vi "TSM Initialise Global (Process Setup).vi"(0 "TSM context":T2, 5 "TestFlowID":string, 9 "configuration file path":string) -> (4 "Initial Configurations":T1, 15 "error out":errorcluster)   [LabVIEW 2019]
uses:
  <vilib>/NI_TestStand_SemiconductorModule/NI_TestStand_Semiconductor_Module.lvlibp/PinMap/General/SemiconductorModuleContext.ctl
  Common/Utility/typedefs/Initial Configurations.ctl
  Common/Instrument Control/DCPower/TSM/TSM SSC DCPower.ctl
  <vilib>/NI_TestStand_SemiconductorModule/NI_TestStand_Semiconductor_Module.lvlibp/PinMap/PinQueryContext/MultiplePinMultipleSessionQueryContext/MultiplePinMultipleSessionQueryContext.lvclass
  Common/Instrument Control/DCPower/SSC DCPower/SSC DCPower.ctl
  Common/Instrument Control/Shared SubVIs/TSM Pin Abstraction/TSM Pin Information.ctl
  Common/Instrument Control/Shared SubVIs/TSM Pin Abstraction/TSM Pin Type Identifier.ctl
  Common/Instrument Control/Shared SubVIs/TSM Pin Abstraction/TSM Expanded Pin Information.ctl
  Common/Instrument Control/Relay/Pin Map/TSM Relay.ctl
  Common/Instrument Control/DAQmx/Pin Map/TSM DAQmx Multi-Task.ctl
  Common/Instrument Control/DAQmx/Pin Map/SSC DAQmx.ctl
  TSM Context Data Access/TSM Context Data Access.lvclass/TSM Context Data Access.ctl
  TSM Context Data Access/Public/Properties/K1 - Write.vi
  TSM Context Data Access/Public/Properties/MODE3 - Write.vi
  TSM Context Data Access/Public/Properties/Z - Write.vi
  TSM Context Data Access/Public/Properties/Y - Write.vi
  TSM Context Data Access/Public/Properties/MODE2 - Write.vi
  TSM Context Data Access/Public/Properties/K1 - Read.vi
  TSM Context Data Access/Public/Properties/MODE3 - Read.vi
  TSM Context Data Access/Public/Properties/MODE2 - Read.vi
  TSM Context Data Access/Public/Properties/Z - Read.vi
  TSM Context Data Access/Public/Properties/Y - Read.vi
  TSM Context Data Access/Public/Properties/S1 - Write .vi
  TSM Context Data Access/Public/Properties/S1 - Read.vi
  TSM Context Data Access/Public/Properties/DNUM - Write.vi
  TSM Context Data Access/Public/Properties/U0 - Write.vi
  TSM Context Data Access/Public/Properties/U1 - Write.vi
  TSM Context Data Access/Public/Properties/U2- Write.vi
  TSM Context Data Access/Public/Properties/U3 - Write.vi
  TSM Context Data Access/Public/Properties/U4 - Write.vi
  TSM Context Data Access/Public/Properties/U5 - Write.vi
  TSM Context Data Access/Public/Properties/U7 - Write.vi
  TSM Context Data Access/Public/Properties/U8 - Write.vi
  TSM Context Data Access/Public/Properties/U9 - Write.vi
  TSM Context Data Access/Public/Properties/Z1 - Write.vi
  TSM Context Data Access/Public/Properties/Z2- Write.vi
  TSM Context Data Access/Public/Properties/Z3 - Write.vi
  TSM Context Data Access/Public/Properties/Z4 - Write.vi
  TSM Context Data Access/Public/Properties/Z5 - Write.vi
  TSM Context Data Access/Public/Properties/Z6 - Write.vi
  TSM Context Data Access/Public/Properties/Z7 - Write.vi
  TSM Context Data Access/Public/Properties/Z8 - Write.vi
  TSM Context Data Access/Public/Properties/Z9 - Write.vi
  TSM Context Data Access/Public/Properties/New_Global/ReferenceData - Write.vi
  TSM Context Data Access/Public/Properties/C1 - Write.vi
  TSM Context Data Access/Public/Properties/C2 - Write.vi
  TSM Context Data Access/Public/Properties/C3 - Write.vi
  TSM Context Data Access/Public/Properties/C4 - Write.vi
  TSM Context Data Access/Public/Properties/C5 - Write.vi
  TSM Context Data Access/Public/Properties/C6 - Write.vi
  TSM Context Data Access/Public/Properties/C7 - Write.vi
  TSM Context Data Access/Public/Properties/C9 - Write.vi
  <vilib>/NI_TestStand_SemiconductorModule/NI_TestStand_Semiconductor_Module.lvlibp/PinMap/Site and Global Data/SetGlobalData.vi
  TSM Context Data Access/Public/Properties/TestFlowID - Write.vi
  <vilib>/NI_TestStand_SemiconductorModule/NI_TestStand_Semiconductor_Module.lvlibp/PinMap/Site and Global Data/GetGlobalData.vi
  <vilib>/NI_TestStand_SemiconductorModule/NI_TestStand_Semiconductor_Module.lvlibp/PinMap/Site and Global Data/SetSiteData.vi
  <vilib>/NI_TestStand_SemiconductorModule/NI_TestStand_Semiconductor_Module.lvlibp
  TSM Context Data Access/TSM Context Data Access.lvclass
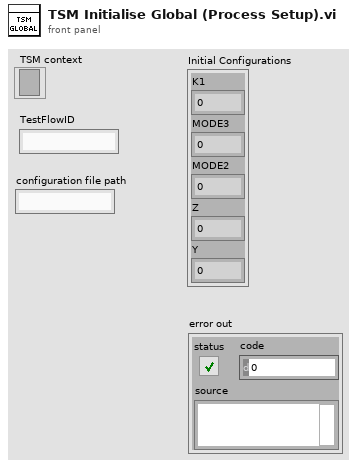
[diagram p1: front panel]
types:
  T1 = typedef "Initial Configurations.ctl" = cluster{"K1":i8, "MODE3":i8, "MODE2":i8, "Z":i8, "Y":i8}
  T2 = typedef "NI_TestStand_Semiconductor_Module.lvlibp/SemiconductorModuleContext.ctl" = refnum<k7>
  T3 = cluster{"unloaded12VRLY":dbl[], "vdiode":dbl[], "RelayDrop":dbl[][], "Initial Configurations":T1}
  T4 = typedef "TSM SSC DCPower.ctl" = cluster{"Pin Query Context":refnum<class "MultiplePinMultipleSessionQueryContext.lvclass">, "SSC":T5[], "Site Numbers":i32[], "Pins":T6[], "Pins Expanded":T8[]}
  T5 = typedef "SSC DCPower.ctl" = cluster{"Session":refnum<k15>, "Chan":string, "Channel List":string}
  T6 = typedef "TSM Pin Information.ctl" = cluster{"Pin":tag, "Type":T7, "Count":i32}
  T7 = typedef "TSM Pin Type Identifier.ctl" = enum8{"DUT Pin", "System Pin", "Pin Group", "Not Determined"}
  T8 = typedef "TSM Expanded Pin Information.ctl" = cluster{"Pin":tag, "Type":T7, "Index":i32}
  T9 = typedef "TSM Relay.ctl" = cluster{"TSM Context":T2, "Relays":tag[]}
  T10 = typedef "TSM DAQmx Multi-Task.ctl" = cluster{"Pin Query Context":refnum<class "MultiplePinMultipleSessionQueryContext.lvclass">, "SSC":T11[], "Site Numbers":i32[]}
  T11 = typedef "SSC DAQmx.ctl" = cluster{"DAQmx Task ":refnum<k21>, "Channels":string, "Channel Lists":string}
  T12 = cluster{"Number Of Sites":i32, "Site Numbers":i32[], "RLY12V_MEAS":T4, "Relays Filtered Pins":string[], "Relay Pin Sessions":T9[], "UDB_EN":T10}
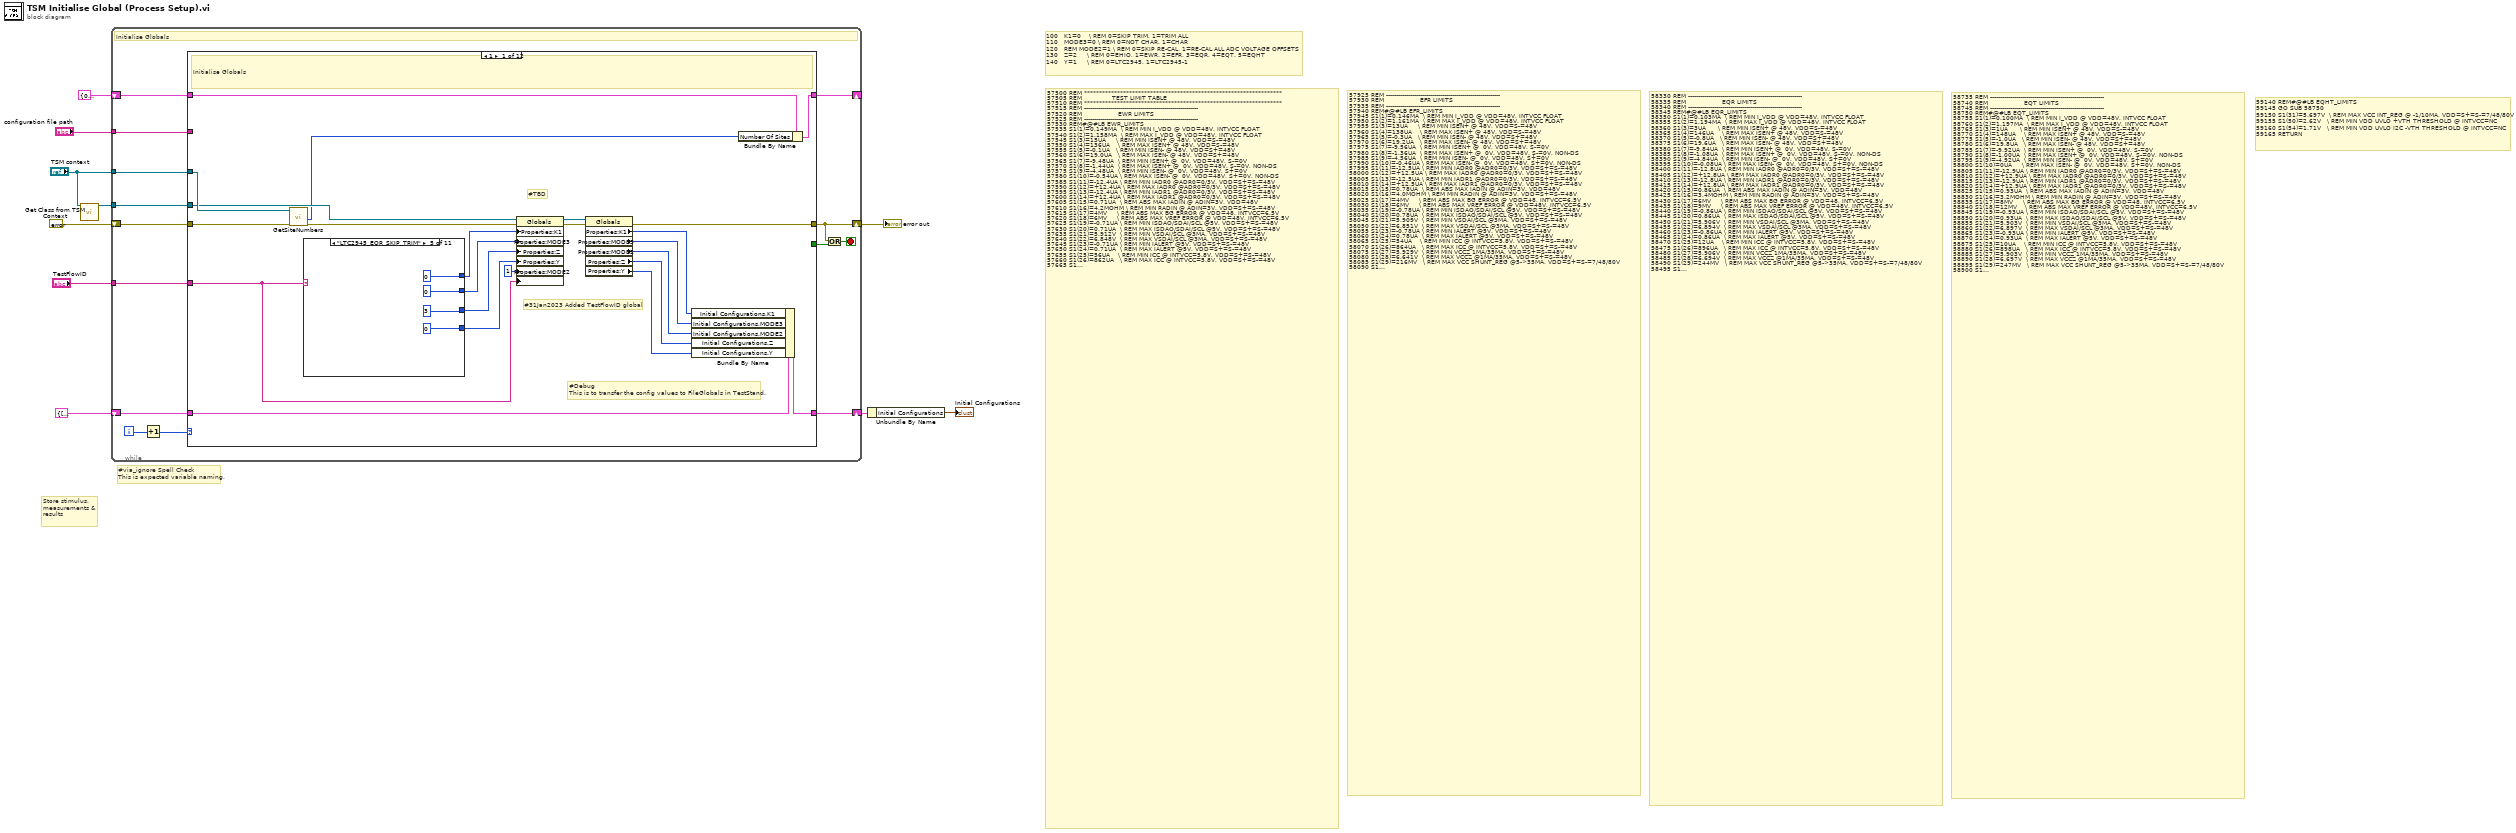
[diagram p0: block diagram]
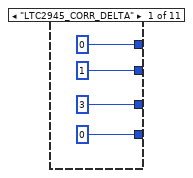
[diagram p2: hidden frame]
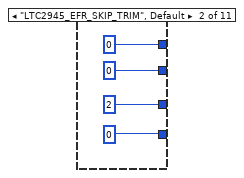
[diagram p3: hidden frame]
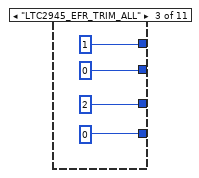
[diagram p4: hidden frame]
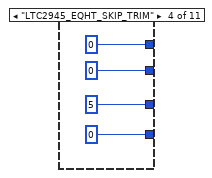
[diagram p5: hidden frame]
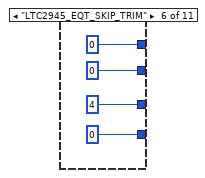
[diagram p6: hidden frame]
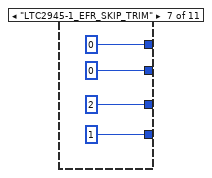
[diagram p7: hidden frame]
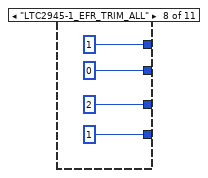
[diagram p8: hidden frame]
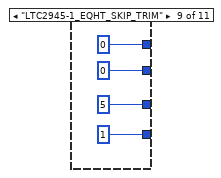
[diagram p9: hidden frame]
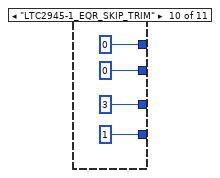
[diagram p10: hidden frame]
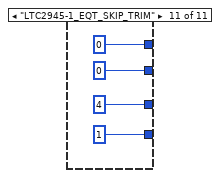
[diagram p11: hidden frame]
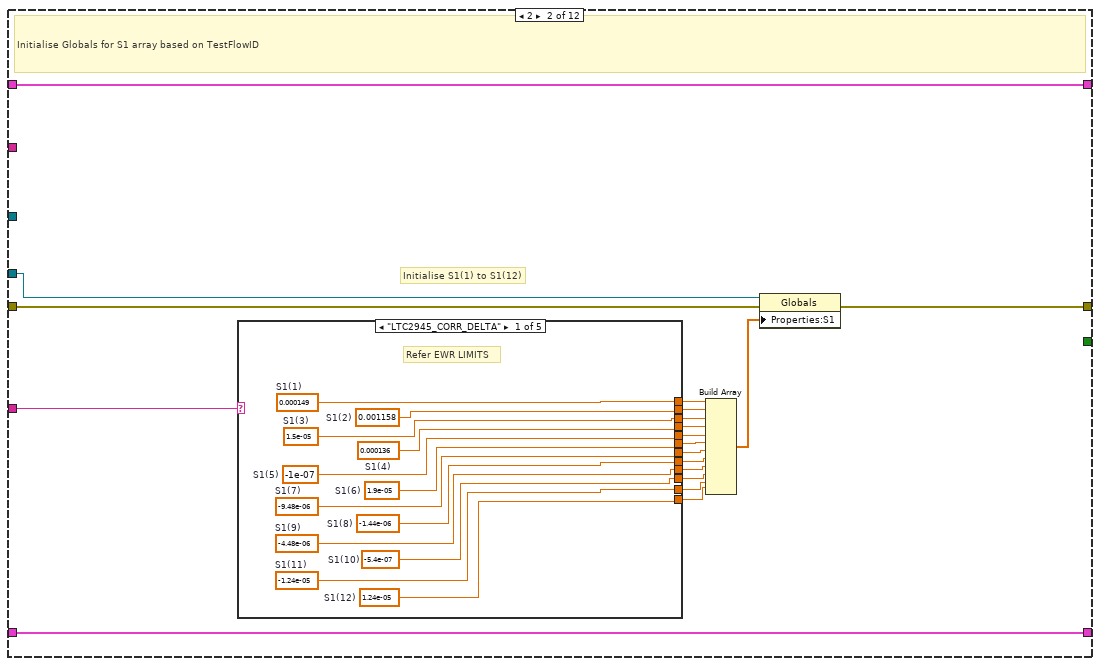
[diagram p12: hidden frame]
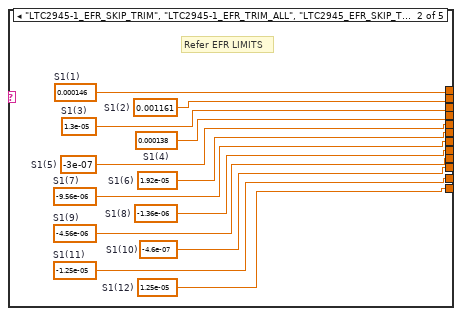
[diagram p13: hidden frame]
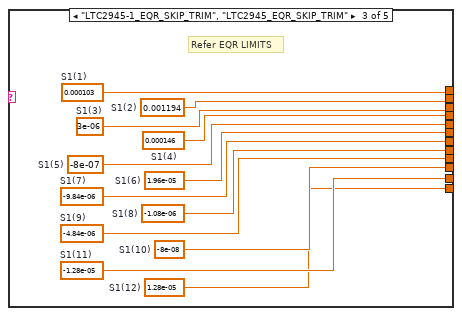
[diagram p14: hidden frame]
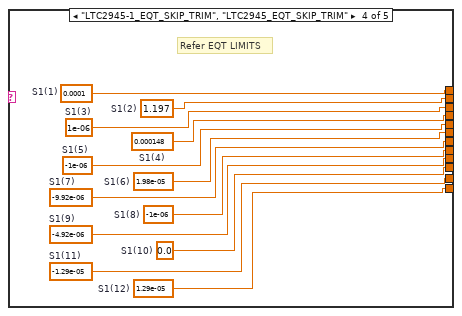
[diagram p15: hidden frame]
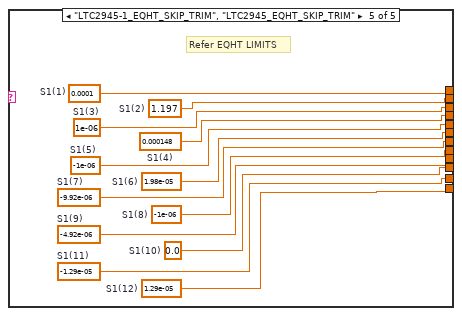
[diagram p16: hidden frame]
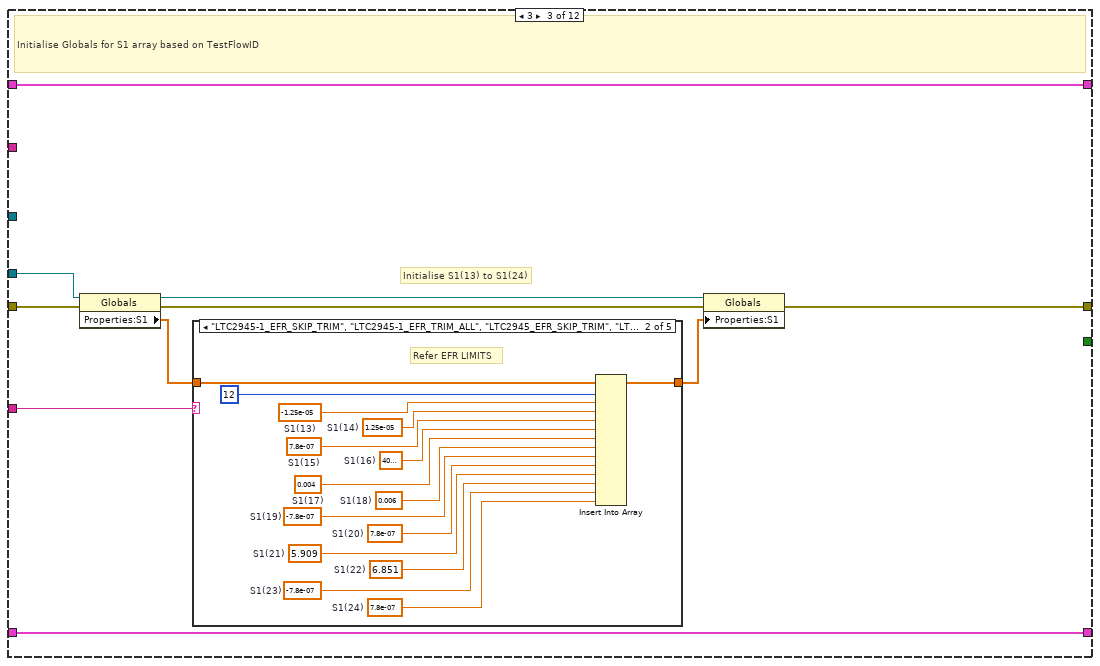
[diagram p17: hidden frame]
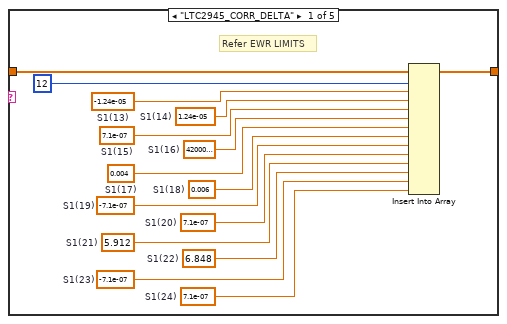
[diagram p18: hidden frame]
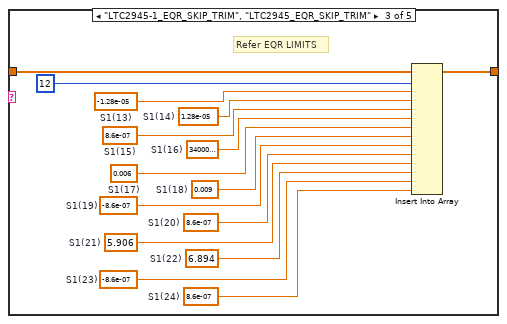
[diagram p19: hidden frame]
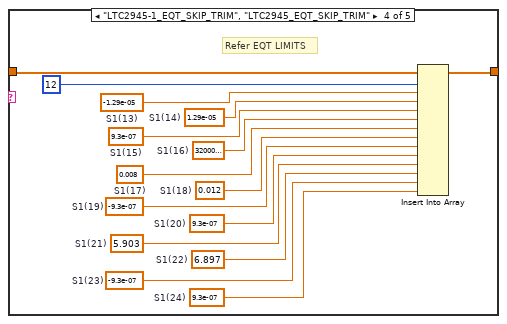
[diagram p20: hidden frame]
diagram:
  # "59140 REM#@#LB EQHT_LIMITS\n59145 GO SUB 58750\n59150 S1(31)=5.697V  \\ REM MAX VCC INT_REG @ -1/10MA, VDD=S+=S-=7/48/80V\n59155 S1(50)=2.62V   \\ REM MIN VDD UVLO +VTH THRESHOLD @ INTVCC=NC\n59160 S1(54)=1.71V   \\ REM MIN VDD UVLO I2C -VTH THRESHOLD @ INTVCC=NC\n59165 RETURN"
  # "58735 REM ---------------------------------------------------------\n58740 REM                  EQT LIMITS\n58745 REM ---------------------------------------------------------\n58750 REM#@#LB EQT_LIMITS\n58755 S1(1)=0.100MA  \\ REM MIN I_VDD @ VDD=48V, INTVCC FLOAT\n58760 S1(2)=1.197MA  \\ REM MAX I_VDD @ VDD=48V, INTVCC FLOAT\n58765 S1(3)=1UA      \\ REM MIN ISEN+ @ 48V, VDD=S-=48V\n58770 S1(4)=148UA    \\ REM MAX ISEN+ @ 48V, VDD=S-=48V\n58775 S1(5)=-1.0UA   \\ REM MIN ISEN- @ 48V, VDD=S+=48V\n58780 S1(6)=19.8UA   \\ REM MAX ISEN- @ 48V, VDD=S+=48V\n58785 S1(7)=-9.92UA  \\ REM MIN ISEN+ @  0V, VDD=48V, S-=0V\n58790 S1(8)=-1.00UA  \\ REM MAX ISEN+ @  0V, VDD=48V, S-=0V, NON-DS\n58795 S1(9)=-4.92UA  \\ REM MIN ISEN- @  0V, VDD=48V, S+=0V\n58800 S1(10)=0UA     \\ REM MAX ISEN- @  0V, VDD=48V, S+=0V, NON-DS\n58805 S1(11)=-12.9UA \\ REM MIN IADR0 @ADR0=0/3V, VDD=S+=S-=48V\n58810 S1(12)=+12.9UA \\ REM MAX IADR0 @ADR0=0/3V, VDD=S+=S-=48V\n58815 S1(13)=-12.9UA \\ REM MIN IADR1 @ADR0=0/3V, VDD=S+=S-=48V\n58820 S1(14)=+12.9UA \\ REM MAX IADR1 @ADR0=0/3V, VDD=S+=S-=48V\n58825 S1(15)=0.93UA  \\ REM ABS MAX IADIN @ ADIN=3V, VDD=48V\n58830 S1(16)=3.2MOHM \\ REM MIN RADIN @ ADIN=3V, VDD=S+=S-=48V\n58835 S1(17)=8MV     \\ REM ABS MAX BG ERROR @ VDD=48, INTVCC=6.5V\n58840 S1(18)=12MV    \\ REM ABS MAX VREF ERROR @ VDD=48V, INTVCC=6.5V\n58845 S1(19)=-0.93UA \\ REM MIN ISDAO/SDAI/SCL @5V, VDD=S+=S-=48V\n58850 S1(20)=0.93UA  \\ REM MAX ISDAO/SDAI/SCL @5V, VDD=S+=S-=48V\n58855 S1(21)=5.903V  \\ REM MIN VSDAI/SCL @3MA, VDD=S+=S-=48V\n58860 S1(22)=6.897V  \\ REM MAX VSDAI/SCL @3MA, VDD=S+=S-=48V\n58865 S1(23)=-0.93UA \\ REM MIN IALERT @5V, VDD=S+=S-=48V\n58870 S1(24)=0.93UA  \\ REM MAX IALERT @5V, VDD=S+=S-=48V\n58875 S1(25)=10UA    \\ REM MIN ICC @ INTVCC=5.8V, VDD=S+=S-=48V\n58880 S1(26)=898UA   \\ REM MAX ICC @ INTVCC=5.8V, VDD=S+=S-=48V\n58885 S1(27)=5.903V  \\ REM MIN VCCZ 1MA/35MA, VDD=S+=S-=48V\n58890 S1(28)=6.697V  \\ REM MAX VCCZ @1MA/35MA, VDD=S+=S-=48V\n58895 S1(29)=247MV   \\ REM MAX VCC SHUNT_REG @5->35MA, VDD=S+=S-=7/48/80V\n58900 S1(30)=4.503V  \\ REM MIN VCC INT_REG @ -1/10MA, VDD=S+=S-=7/48/80V\n58905 S1(31)=5.497V  \\ REM MAX VCC INT_REG @ -1/10MA, VDD=S+=S-=7/48/80V\n58910 S1(32)=198MV   \\ REM MAX VCC LOAD REG @1->10MA, VDD=S+=S-=7/48/80V\n58915 S1(33)=1.92UA  \\ REM MAX ISEN+ SHDN @ 0/48V, VDD=S-=48V\n58920 S1(34)=0.92UA  \\ REM MAX ISEN- SHDN @ 0/48V, VDD=48V, S-=0V\n58925 S1(35)=79UA    \\ REM MAX ICC_SD @ INTVCC=5V, VDD=S+=S-=48V\n58930 S1(36)=69UA    \\ REM MAX IDD_SD @ INTVCC=NC, S+=S-=48V\n58935 S1(37)=0.73%   \\ REM ABS MAX ADC DELTA VSENSE T.U.E, VDD=4/48/80V\n58940 S1(38)=0.73%   \\ REM ABS MAX ADC ADIN T.U.E, VDD=4/48/80V, S+=48V\n58945 S1(39)=0.73%   \\ REM ABS MAX ADC VIN (VDD&S+) T.U.E, S+=48V\n58950 S1(40)=1.92V   \\ REM MIN ADR0/AD1 VIH @ VDD=48V\n58955 S1(41)=2.68V   \\ REM MAX ADR0/AD1 VIH @ VDD=48V\n58960 S1(42)=0.32V   \\ REM MIN ADR0/AD1 VIL @ VDD=48V\n58965 S1(43)=0.88V   \\ REM MAX ADR0/AD1 VIL @ VDD=48V\n58970 S1(44)=10MV    \\ REM MIN SDAO/ALERT VOL @8MA, VDD=48V\n58975 S1(45)=398MV   \\ REM MAX SDAO/ALERT VOL @8MA, VDD=48V\n58980 S1(46)=1.52V   \\ REM MIN SDAI/SCL VTH @ VDD=48V\n58985 S1(47)=2.18V   \\ REM MAX SDAI/SCL VTH @ VDD=48V\n58990 S1(48)=2.31V   \\ REM MIN VCC UVLO +VTH THRESHOLD @ VDD=INTVCC\n58995 S1(49)=2.68V   \\ REM MAX VCC UVLO +VTH THRESHOLD @ VDD=INTVCC\n59000 S1(50)=2.92V   \\ REM MIN VDD UVLO +VTH THRESHOLD @ INTVCC=NC\n59005 S1(51)=3.48V   \\ REM MAX VDD UVLO +VTH THRESHOLD @ INTVCC=NC\n59010 S1(52)=1.51V   \\ REM MIN VCC UVLO I2C -VTH THRESHOLD @ VDD=INTVCC\n59015 S1(53)=2.60V   \\ REM MAX VCC UVLO I2C +VTH THRESHOLD @ VDD=INTVCC (NON-DS)\n59020 S1(54)=2.01V   \\ REM MIN VDD UVLO I2C -VTH THRESHOLD @ INTVCC=NC\n59025 S1(55)=3.20V   \\ REM MAX VDD UVLO I2C +VTH THRESHOLD @ INTVCC=NC, (NON-DS)\n59030 S1(59)=25MS    \\ REM STUCK BUS MIN TIMING\n59035 S1(60)=50MS    \\ REM STUCK BUS MAX TIMING\n59040 S1(61)=0.20MA  \\ REM MIN ABSMAX I_VDD @ VDD=90/100V\n59045 S1(62)=2.00MA  \\ REM MAX ABSMAX I_VDD @ VDD=90/100V\n59050 S1(63)=1UA     \\ REM MIN ABSMAX ISEN+ @ VSEN+=100V\n59055 S1(64)=200UA   \\ REM MAX ABSMAX ISEN+ @ VSEN+=100V\n59060 S1(65)=-0.2UA  \\ REM MIN ABSMAX ISEN- @ VSEN-=100V\n59065 S1(66)=40UA    \\ REM MAX ABSMAX ISEN- @ VSEN-=100V\n59070 S1(67)=2.99LSB \\ REM ABS MAX ADC DELTA VSENSE INL ERROR, VDD=2.7V\n59075 S1(68)=1.99LSB \\ REM ABS MAX ADC ADIN INL ERROR, VDD=4/48/80V, S+=48V\n59080 S1(69)=1.99LSB \\ REM ABS MAX ADC VIN (VDD&S+) INL ERROR, S+=48V\n59085 S1(70)=3.09LSB \\ REM ABS MAX ADC DELTA VSENSE VOS, VDD=2.7V\n59090 S1(71)=1.09LSB \\ REM ABS MAX ADC ADIN VOS, VDD=2.7V\n59095 S1(72)=1.49LSB \\ REM ABS MAX ADC VIN (VDD&S+) VOS, S+=48V\n59100 S1(73)=30.01MS \\ REM MIN VIN/ADIN CONVERSION TIME @ VDD=S+=S-=48V\n59105 S1(74)=35.99MS \\ REM MAX VIN/ADIN CONVERSION TIME @ VDD=S+=S-=48V\n59110 S1(75)=60.02MS \\ REM MIN DVSENSE CONVERSION TIME @ VDD=S+=S-=48V\n59115 S1(76)=71.98MS \\ REM MAX DVSENSE CONVERSION TIME @ VDD=S+=S-=48V\n59120 S1(77)=6.01HZ  \\ REM MIN CONVERSION RATE @ VDD=S+=S-=48V\n59125 S1(78)=8.99HZ  \\ REM MAX CONVERSION RATE @ VDD=S+=S-=48V\n59130 Z0=1\n59135 RETURN"
  # "58330 REM ---------------------------------------------------------\n58335 REM                  EQR LIMITS\n58340 REM ---------------------------------------------------------\n58345 REM#@#LB EQR_LIMITS\n58350 S1(1)=0.103MA  \\ REM MIN I_VDD @ VDD=48V, INTVCC FLOAT\n58355 S1(2)=1.194MA  \\ REM MAX I_VDD @ VDD=48V, INTVCC FLOAT\n58360 S1(3)=3UA      \\ REM MIN ISEN+ @ 48V, VDD=S-=48V\n58365 S1(4)=146UA    \\ REM MAX ISEN+ @ 48V, VDD=S-=48V\n58370 S1(5)=-0.8UA   \\ REM MIN ISEN- @ 48V, VDD=S+=48V\n58375 S1(6)=19.6UA   \\ REM MAX ISEN- @ 48V, VDD=S+=48V\n58380 S1(7)=-9.84UA  \\ REM MIN ISEN+ @  0V, VDD=48V, S-=0V\n58385 S1(8)=-1.08UA  \\ REM MAX ISEN+ @  0V, VDD=48V, S-=0V, NON-DS\n58390 S1(9)=-4.84UA  \\ REM MIN ISEN- @  0V, VDD=48V, S+=0V\n58395 S1(10)=-0.08UA \\ REM MAX ISEN- @  0V, VDD=48V, S+=0V, NON-DS\n58400 S1(11)=-12.8UA \\ REM MIN IADR0 @ADR0=0/3V, VDD=S+=S-=48V\n58405 S1(12)=+12.8UA \\ REM MAX IADR0 @ADR0=0/3V, VDD=S+=S-=48V\n58410 S1(13)=-12.8UA \\ REM MIN IADR1 @ADR0=0/3V, VDD=S+=S-=48V\n58415 S1(14)=+12.8UA \\ REM MAX IADR1 @ADR0=0/3V, VDD=S+=S-=48V\n58420 S1(15)=0.86UA  \\ REM ABS MAX IADIN @ ADIN=3V, VDD=48V\n58425 S1(16)=3.4MOHM \\ REM MIN RADIN @ ADIN=3V, VDD=S+=S-=48V\n58430 S1(17)=6MV     \\ REM ABS MAX BG ERROR @ VDD=48, INTVCC=6.5V\n58435 S1(18)=9MV     \\ REM ABS MAX VREF ERROR @ VDD=48V, INTVCC=6.5V\n58440 S1(19)=-0.86UA \\ REM MIN ISDAO/SDAI/SCL @5V, VDD=S+=S-=48V\n58445 S1(20)=0.86UA  \\ REM MAX ISDAO/SDAI/SCL @5V, VDD=S+=S-=48V\n58450 S1(21)=5.906V  \\ REM MIN VSDAI/SCL @3MA, VDD=S+=S-=48V\n58455 S1(22)=6.894V  \\ REM MAX VSDAI/SCL @3MA, VDD=S+=S-=48V\n58460 S1(23)=-0.86UA \\ REM MIN IALERT @5V, VDD=S+=S-=48V\n58465 S1(24)=0.86UA  \\ REM MAX IALERT @5V, VDD=S+=S-=48V\n58470 S1(25)=12UA    \\ REM MIN ICC @ INTVCC=5.8V, VDD=S+=S-=48V\n58475 S1(26)=896UA   \\ REM MAX ICC @ INTVCC=5.8V, VDD=S+=S-=48V\n58480 S1(27)=5.906V  \\ REM MIN VCCZ 1MA/35MA, VDD=S+=S-=48V\n58485 S1(28)=6.694V  \\ REM MAX VCCZ @1MA/35MA, VDD=S+=S-=48V\n58490 S1(29)=244MV   \\ REM MAX VCC SHUNT_REG @5->35MA, VDD=S+=S-=7/48/80V\n58495 S1(30)=4.506V  \\ REM MIN VCC INT_REG @ -1/10MA, VDD=S+=S-=7/48/80V\n58500 S1(31)=5.494V  \\ REM MAX VCC INT_REG @ -1/10MA, VDD=S+=S-=7/48/80V\n58505 S1(32)=196MV   \\ REM MAX VCC LOAD REG @1->10MA, VDD=S+=S-=7/48/80V\n58510 S1(33)=1.88UA  \\ REM MAX ISEN+ SHDN @ 0/48V, VDD=S-=48V\n58515 S1(34)=0.88UA  \\ REM MAX ISEN- SHDN @ 0/48V, VDD=48V, S-=0V\n58520 S1(35)=77UA    \\ REM MAX ICC_SD @ INTVCC=5V, VDD=S+=S-=48V\n58525 S1(36)=67UA    \\ REM MAX IDD_SD @ INTVCC=NC, S+=S-=48V\n58530 S1(37)=0.71%   \\ REM ABS MAX ADC DELTA VSENSE T.U.E, VDD=4/48/80V\n58535 S1(38)=0.71%   \\ REM ABS MAX ADC ADIN T.U.E, VDD=4/48/80V, S+=48V\n58540 S1(39)=0.71%   \\ REM ABS MAX ADC VIN (VDD&S+) T.U.E, S+=48V\n58545 S1(40)=1.94V   \\ REM MIN ADR0/AD1 VIH @ VDD=48V\n58550 S1(41)=2.66V   \\ REM MAX ADR0/AD1 VIH @ VDD=48V\n58555 S1(42)=0.34V   \\ REM MIN ADR0/AD1 VIL @ VDD=48V\n58560 S1(43)=0.86V   \\ REM MAX ADR0/AD1 VIL @ VDD=48V\n58565 S1(44)=12MV    \\ REM MIN SDAO/ALERT VOL @8MA, VDD=48V\n58570 S1(45)=396MV   \\ REM MAX SDAO/ALERT VOL @8MA, VDD=48V\n58575 S1(46)=1.54V   \\ REM MIN SDAI/SCL VTH @ VDD=48V\n58580 S1(47)=2.16V   \\ REM MAX SDAI/SCL VTH @ VDD=48V\n58585 S1(48)=2.32V   \\ REM MIN VCC UVLO +VTH THRESHOLD @ VDD=INTVCC\n58590 S1(49)=2.67V   \\ REM MAX VCC UVLO +VTH THRESHOLD @ VDD=INTVCC\n58595 S1(50)=2.94V   \\ REM MIN VDD UVLO +VTH THRESHOLD @ INTVCC=NC\n58600 S1(51)=3.46V   \\ REM MAX VDD UVLO +VTH THRESHOLD @ INTVCC=NC\n58605 S1(52)=1.52V   \\ REM MIN VCC UVLO I2C -VTH THRESHOLD @ VDD=INTVCC\n58610 S1(53)=2.59V   \\ REM MAX VCC UVLO I2C +VTH THRESHOLD @ VDD=INTVCC (NON-DS)\n58615 S1(54)=2.02V   \\ REM MIN VDD UVLO I2C -VTH THRESHOLD @ INTVCC=NC\n58620 S1(55)=3.19V   \\ REM MAX VDD UVLO I2C +VTH THRESHOLD @ INTVCC=NC, (NON-DS)\n58625 S1(59)=25MS    \\ REM STUCK BUS MIN TIMING\n58630 S1(60)=50MS    \\ REM STUCK BUS MAX TIMING\n58635 S1(61)=0.21MA  \\ REM MIN ABSMAX I_VDD @ VDD=90/100V\n58640 S1(62)=1.99MA  \\ REM MAX ABSMAX I_VDD @ VDD=90/100V\n58645 S1(63)=3UA     \\ REM MIN ABSMAX ISEN+ @ VSEN+=100V\n58650 S1(64)=198UA   \\ REM MAX ABSMAX ISEN+ @ VSEN+=100V\n58655 S1(65)=0UA     \\ REM MIN ABSMAX ISEN- @ VSEN-=100V\n58660 S1(66)=39.8UA  \\ REM MAX ABSMAX ISEN- @ VSEN-=100V\n58665 S1(67)=2.98LSB \\ REM ABS MAX ADC DELTA VSENSE INL ERROR, VDD=2.7V\n58670 S1(68)=1.98LSB \\ REM ABS MAX ADC ADIN INL ERROR, VDD=4/48/80V, S+=48V\n58675 S1(69)=1.98LSB \\ REM ABS MAX ADC VIN (VDD&S+) INL ERROR, S+=48V\n58680 S1(70)=3.08LSB \\ REM ABS MAX ADC DELTA VSENSE VOS, VDD=2.7V\n58685 S1(71)=1.08LSB \\ REM ABS MAX ADC ADIN VOS, VDD=2.7V\n58690 S1(72)=1.48LSB \\ REM ABS MAX ADC VIN (VDD&S+) VOS, S+=48V\n58695 S1(73)=30.02MS \\ REM MIN VIN/ADIN CONVERSION TIME @ VDD=S+=S-=48V\n58700 S1(74)=35.98MS \\ REM MAX VIN/ADIN CONVERSION TIME @ VDD=S+=S-=48V\n58705 S1(75)=60.04MS \\ REM MIN DVSENSE CONVERSION TIME @ VDD=S+=S-=48V\n58710 S1(76)=71.96MS \\ REM MAX DVSENSE CONVERSION TIME @ VDD=S+=S-=48V\n58715 S1(77)=6.02HZ  \\ REM MIN CONVERSION RATE @ VDD=S+=S-=48V\n58720 S1(78)=8.98HZ  \\ REM MAX CONVERSION RATE @ VDD=S+=S-=48V\n58725 Z0=1\n58730 RETURN"
  # "57925 REM ---------------------------------------------------------\n57930 REM                  EFR LIMITS\n57935 REM ---------------------------------------------------------\n57940 REM#@#LB EFR_LIMITS\n57945 S1(1)=0.146MA  \\ REM MIN I_VDD @ VDD=48V, INTVCC FLOAT\n57950 S1(2)=1.161MA  \\ REM MAX I_VDD @ VDD=48V, INTVCC FLOAT\n57955 S1(3)=13UA     \\ REM MIN ISEN+ @ 48V, VDD=S-=48V\n57960 S1(4)=138UA    \\ REM MAX ISEN+ @ 48V, VDD=S-=48V\n57965 S1(5)=-0.3UA   \\ REM MIN ISEN- @ 48V, VDD=S+=48V\n57970 S1(6)=19.2UA   \\ REM MAX ISEN- @ 48V, VDD=S+=48V\n57975 S1(7)=-9.56UA  \\ REM MIN ISEN+ @  0V, VDD=48V, S-=0V\n57980 S1(8)=-1.36UA  \\ REM MAX ISEN+ @  0V, VDD=48V, S-=0V, NON-DS\n57985 S1(9)=-4.56UA  \\ REM MIN ISEN- @  0V, VDD=48V, S+=0V\n57990 S1(10)=-0.46UA \\ REM MAX ISEN- @  0V, VDD=48V, S+=0V, NON-DS\n57995 S1(11)=-12.5UA \\ REM MIN IADR0 @ADR0=0/3V, VDD=S+=S-=48V\n58000 S1(12)=+12.5UA \\ REM MAX IADR0 @ADR0=0/3V, VDD=S+=S-=48V\n58005 S1(13)=-12.5UA \\ REM MIN IADR1 @ADR0=0/3V, VDD=S+=S-=48V\n58010 S1(14)=+12.5UA \\ REM MAX IADR1 @ADR0=0/3V, VDD=S+=S-=48V\n58015 S1(15)=0.78UA  \\ REM ABS MAX IADIN @ ADIN=3V, VDD=48V\n58020 S1(16)=4.0MOHM \\ REM MIN RADIN @ ADIN=3V, VDD=S+=S-=48V\n58025 S1(17)=4MV     \\ REM ABS MAX BG ERROR @ VDD=48, INTVCC=6.5V\n58030 S1(18)=6MV     \\ REM ABS MAX VREF ERROR @ VDD=48V, INTVCC=6.5V\n58035 S1(19)=-0.78UA \\ REM MIN ISDAO/SDAI/SCL @5V, VDD=S+=S-=48V\n58040 S1(20)=0.78UA  \\ REM MAX ISDAO/SDAI/SCL @5V, VDD=S+=S-=48V\n58045 S1(21)=5.909V  \\ REM MIN VSDAI/SCL @3MA, VDD=S+=S-=48V\n58050 S1(22)=6.851V  \\ REM MAX VSDAI/SCL @3MA, VDD=S+=S-=48V\n58055 S1(23)=-0.78UA \\ REM MIN IALERT @5V, VDD=S+=S-=48V\n58060 S1(24)=0.78UA  \\ REM MAX IALERT @5V, VDD=S+=S-=48V\n58065 S1(25)=54UA    \\ REM MIN ICC @ INTVCC=5.8V, VDD=S+=S-=48V\n58070 S1(26)=864UA   \\ REM MAX ICC @ INTVCC=5.8V, VDD=S+=S-=48V\n58075 S1(27)=5.929V  \\ REM MIN VCCZ 1MA/35MA, VDD=S+=S-=48V\n58080 S1(28)=6.641V  \\ REM MAX VCCZ @1MA/35MA, VDD=S+=S-=48V\n58085 S1(29)=216MV   \\ REM MAX VCC SHUNT_REG @5->35MA, VDD=S+=S-=7/48/80V\n58090 S1(30)=4.769V  \\ REM MIN VCC INT_REG @ -1/10MA, VDD=S+=S-=7/48/80V\n58095 S1(31)=5.261V  \\ REM MAX VCC INT_REG @ -1/10MA, VDD=S+=S-=7/48/80V\n58100 S1(32)=182MV   \\ REM MAX VCC LOAD REG @1->10MA, VDD=S+=S-=7/48/80V\n58105 S1(33)=1.74UA  \\ REM MAX ISEN+ SHDN @ 0/48V, VDD=S-=48V\n58110 S1(34)=0.83UA  \\ REM MAX ISEN- SHDN @ 0/48V, VDD=48V, S-=0V\n58115 S1(35)=37UA    \\ REM MAX ICC_SD @ INTVCC=5V, VDD=S+=S-=48V\n58120 S1(36)=64UA    \\ REM MAX IDD_SD @ INTVCC=NC, S+=S-=48V\n58125 S1(37)=0.54%   \\ REM ABS MAX ADC DELTA VSENSE T.U.E, VDD=4/48/80V\n58130 S1(38)=0.54%   \\ REM ABS MAX ADC ADIN T.U.E, VDD=4/48/80V, S+=48V\n58135 S1(39)=0.54%   \\ REM ABS MAX ADC VIN (VDD&S+) T.U.E, S+=48V\n58140 S1(40)=1.98V   \\ REM MIN ADR0/AD1 VIH @ VDD=48V\n58145 S1(41)=2.62V   \\ REM MAX ADR0/AD1 VIH @ VDD=48V\n58150 S1(42)=0.38V   \\ REM MIN ADR0/AD1 VIL @ VDD=48V\n58155 S1(43)=0.82V   \\ REM MAX ADR0/AD1 VIL @ VDD=48V\n58160 S1(44)=84MV    \\ REM MIN SDAO/ALERT VOL @8MA, VDD=48V\n58165 S1(45)=324MV   \\ REM MAX SDAO/ALERT VOL @8MA, VDD=48V\n58170 S1(46)=1.57V   \\ REM MIN SDAI/SCL VTH @ VDD=48V\n58175 S1(47)=2.13V   \\ REM MAX SDAI/SCL VTH @ VDD=48V\n58180 S1(48)=2.34V   \\ REM MIN VCC UVLO +VTH THRESHOLD @ VDD=INTVCC\n58185 S1(49)=2.65V   \\ REM MAX VCC UVLO +VTH THRESHOLD @ VDD=INTVCC\n58190 S1(50)=3.06V   \\ REM MIN VDD UVLO +VTH THRESHOLD @ INTVCC=NC\n58195 S1(51)=3.32V   \\ REM MAX VDD UVLO +VTH THRESHOLD @ INTVCC=NC\n58200 S1(52)=1.65V   \\ REM MIN VCC UVLO I2C -VTH THRESHOLD @ VDD=INTVCC\n58205 S1(53)=2.46V   \\ REM MAX VCC UVLO I2C +VTH THRESHOLD @ VDD=INTVCC (NON-DS)\n58210 S1(54)=2.18V   \\ REM MIN VDD UVLO I2C -VTH THRESHOLD @ INTVCC=NC\n58215 S1(55)=3.03V   \\ REM MAX VDD UVLO I2C +VTH THRESHOLD @ INTVCC=NC, (NON-DS)\n58220 S1(59)=25MS    \\ REM STUCK BUS MIN TIMING\n58225 S1(60)=50MS    \\ REM STUCK BUS MAX TIMING\n58230 S1(61)=0.26MA  \\ REM MIN ABSMAX I_VDD @ VDD=90/100V\n58235 S1(62)=1.96MA  \\ REM MAX ABSMAX I_VDD @ VDD=90/100V\n58240 S1(63)=13UA    \\ REM MIN ABSMAX ISEN+ @ VSEN+=100V\n58245 S1(64)=190UA   \\ REM MAX ABSMAX ISEN+ @ VSEN+=100V\n58250 S1(65)=0.4UA   \\ REM MIN ABSMAX ISEN- @ VSEN-=100V\n58255 S1(66)=39.4UA  \\ REM MAX ABSMAX ISEN- @ VSEN-=100V\n58260 S1(67)=2.97LSB \\ REM ABS MAX ADC DELTA VSENSE INL ERROR, VDD=2.7V\n58265 S1(68)=1.97LSB \\ REM ABS MAX ADC ADIN INL ERROR, VDD=4/48/80V, S+=48V\n58270 S1(69)=1.97LSB \\ REM ABS MAX ADC VIN (VDD&S+) INL ERROR, S+=48V\n58275 S1(70)=3.07LSB \\ REM ABS MAX ADC DELTA VSENSE VOS, VDD=2.7V\n58280 S1(71)=1.07LSB \\ REM ABS MAX ADC ADIN VOS, VDD=2.7V\n58285 S1(72)=1.47LSB \\ REM ABS MAX ADC VIN (VDD&S+) VOS, S+=48V\n58290 S1(73)=30.05MS \\ REM MIN VIN/ADIN CONVERSION TIME @ VDD=S+=S-=48V\n58295 S1(74)=35.91MS \\ REM MAX VIN/ADIN CONVERSION TIME @ VDD=S+=S-=48V\n58300 S1(75)=60.10MS \\ REM MIN DVSENSE CONVERSION TIME @ VDD=S+=S-=48V\n58305 S1(76)=71.84MS \\ REM MAX DVSENSE CONVERSION TIME @ VDD=S+=S-=48V\n58310 S1(77)=6.05HZ  \\ REM MIN CONVERSION RATE @ VDD=S+=S-=48V\n58315 S1(78)=8.95HZ  \\ REM MAX CONVERSION RATE @ VDD=S+=S-=48V\n58320 Z0=1\n58325 RETURN"
  # "57500 REM ******************************************************************\n57505 REM               TEST LIMIT TABLE\n57510 REM ******************************************************************\n57515 REM ---------------------------------------------------------\n57520 REM                  EWR LIMITS\n57525 REM ---------------------------------------------------------\n57530 REM#@#LB EWR_LIMITS\n57535 S1(1)=0.149MA  \\ REM MIN I_VDD @ VDD=48V, INTVCC FLOAT\n57540 S1(2)=1.158MA  \\ REM MAX I_VDD @ VDD=48V, INTVCC FLOAT\n57545 S1(3)=15UA     \\ REM MIN ISEN+ @ 48V, VDD=S-=48V\n57550 S1(4)=136UA    \\ REM MAX ISEN+ @ 48V, VDD=S-=48V\n57555 S1(5)=-0.1UA   \\ REM MIN ISEN- @ 48V, VDD=S+=48V\n57560 S1(6)=19.0UA   \\ REM MAX ISEN- @ 48V, VDD=S+=48V\n57565 S1(7)=-9.48UA  \\ REM MIN ISEN+ @  0V, VDD=48V, S-=0V\n57570 S1(8)=-1.44UA  \\ REM MAX ISEN+ @  0V, VDD=48V, S-=0V, NON-DS\n57575 S1(9)=-4.48UA  \\ REM MIN ISEN- @  0V, VDD=48V, S+=0V\n57580 S1(10)=-0.54UA \\ REM MAX ISEN- @  0V, VDD=48V, S+=0V, NON-DS\n57585 S1(11)=-12.4UA \\ REM MIN IADR0 @ADR0=0/3V, VDD=S+=S-=48V\n57590 S1(12)=+12.4UA \\ REM MAX IADR0 @ADR0=0/3V, VDD=S+=S-=48V\n57595 S1(13)=-12.4UA \\ REM MIN IADR1 @ADR0=0/3V, VDD=S+=S-=48V\n57600 S1(14)=+12.4UA \\ REM MAX IADR1 @ADR0=0/3V, VDD=S+=S-=48V\n57605 S1(15)=0.71UA  \\ REM ABS MAX IADIN @ ADIN=3V, VDD=48V\n57610 S1(16)=4.2MOHM \\ REM MIN RADIN @ ADIN=3V, VDD=S+=S-=48V\n57615 S1(17)=4MV     \\ REM ABS MAX BG ERROR @ VDD=48, INTVCC=6.5V\n57620 S1(18)=6MV     \\ REM ABS MAX VREF ERROR @ VDD=48V, INTVCC=6.5V\n57625 S1(19)=-0.71UA \\ REM MIN ISDAO/SDAI/SCL @5V, VDD=S+=S-=48V\n57630 S1(20)=0.71UA  \\ REM MAX ISDAO/SDAI/SCL @5V, VDD=S+=S-=48V\n57635 S1(21)=5.912V  \\ REM MIN VSDAI/SCL @3MA, VDD=S+=S-=48V\n57640 S1(22)=6.848V  \\ REM MAX VSDAI/SCL @3MA, VDD=S+=S-=48V\n57645 S1(23)=-0.71UA \\ REM MIN IALERT @5V, VDD=S+=S-=48V\n57650 S1(24)=0.71UA  \\ REM MAX IALERT @5V, VDD=S+=S-=48V\n57655 S1(25)=56UA    \\ REM MIN ICC @ INTVCC=5.8V, VDD=S+=S-=48V\n57660 S1(26)=862UA   \\ REM MAX ICC @ INTVCC=5.8V, VDD=S+=S-=48V\n57665 S1(27)=5.932V  \\ REM MIN VCCZ 1MA/35MA, VDD=S+=S-=48V\n57670 S1(28)=6.638V  \\ REM MAX VCCZ @1MA/35MA, VDD=S+=S-=48V\n57675 S1(29)=213MV   \\ REM MAX VCC SHUNT_REG @5->35MA, VDD=S+=S-=7/48/80V\n57680 S1(30)=4.772V  \\ REM MIN VCC INT_REG @ -1/10MA, VDD=S+=S-=7/48/80V\n57685 S1(31)=5.258V  \\ REM MAX VCC INT_REG @ -1/10MA, VDD=S+=S-=7/48/80V\n57690 S1(32)=180MV   \\ REM MAX VCC LOAD REG @1->10MA, VDD=S+=S-=7/48/80V\n57695 S1(33)=1.70UA  \\ REM MAX ISEN+ SHDN @ 0/48V, VDD=S-=48V\n57700 S1(34)=0.79UA  \\ REM MAX ISEN- SHDN @ 0/48V, VDD=48V, S-=0V\n57705 S1(35)=35UA    \\ REM MAX ICC_SD @ INTVCC=5V, VDD=S+=S-=48V\n57710 S1(36)=63UA    \\ REM MAX IDD_SD @ INTVCC=NC, S+=S-=48V\n57715 S1(37)=0.52%   \\ REM ABS MAX ADC DELTA VSENSE T.U.E, VDD=4/48/80V\n57720 S1(38)=0.52%   \\ REM ABS MAX ADC ADIN T.U.E, VDD=4/48/80V, S+=48V\n57725 S1(39)=0.52%   \\ REM ABS MAX ADC VIN (VDD&S+) T.U.E, S+=48V\n57730 S1(40)=2.0V    \\ REM MIN ADR0/AD1 VIH @ VDD=48V\n57735 S1(41)=2.6V    \\ REM MAX ADR0/AD1 VIH @ VDD=48V\n57740 S1(42)=0.40V   \\ REM MIN ADR0/AD1 VIL @ VDD=48V\n57745 S1(43)=0.80V   \\ REM MAX ADR0/AD1 VIL @ VDD=48V\n57750 S1(44)=86MV    \\ REM MIN SDAO/ALERT VOL @8MA, VDD=48V\n57755 S1(45)=322MV   \\ REM MAX SDAO/ALERT VOL @8MA, VDD=48V\n57760 S1(46)=1.59V   \\ REM MIN SDAI/SCL VTH @ VDD=48V\n57765 S1(47)=2.11V   \\ REM MAX SDAI/SCL VTH @ VDD=48V\n57770 S1(48)=2.35V   \\ REM MIN VCC UVLO +VTH THRESHOLD @ VDD=INTVCC\n57775 S1(49)=2.64V   \\ REM MAX VCC UVLO +VTH THRESHOLD @ VDD=INTVCC\n57780 S1(50)=3.08V   \\ REM MIN VDD UVLO +VTH THRESHOLD @ INTVCC=NC\n57785 S1(51)=3.30V   \\ REM MAX VDD UVLO +VTH THRESHOLD @ INTVCC=NC\n57790 S1(52)=1.66V   \\ REM MIN VCC UVLO I2C -VTH THRESHOLD @ VDD=INTVCC\n57795 S1(53)=2.45V   \\ REM MAX VCC UVLO I2C +VTH THRESHOLD @ VDD=INTVCC (NON-DS)\n57800 S1(54)=2.19V   \\ REM MIN VDD UVLO I2C -VTH THRESHOLD @ INTVCC=NC\n57805 S1(55)=3.02V   \\ REM MAX VDD UVLO I2C +VTH THRESHOLD @ INTVCC=NC, (NON-DS)\n57810 S1(59)=25MS    \\ REM STUCK BUS MIN TIMING\n57815 S1(60)=50MS    \\ REM STUCK BUS MAX TIMING\n57820 S1(61)=0.27MA  \\ REM MIN ABSMAX I_VDD @ VDD=90/100V\n57825 S1(62)=1.95MA  \\ REM MAX ABSMAX I_VDD @ VDD=90/100V\n57830 S1(63)=15UA    \\ REM MIN ABSMAX ISEN+ @ VSEN+=100V\n57835 S1(64)=188UA   \\ REM MAX ABSMAX ISEN+ @ VSEN+=100V\n57840 S1(65)=0.6UA   \\ REM MIN ABSMAX ISEN- @ VSEN-=100V\n57845 S1(66)=39.2UA  \\ REM MAX ABSMAX ISEN- @ VSEN-=100V\n57850 S1(67)=2.96LSB \\ REM ABS MAX ADC DELTA VSENSE INL ERROR, VDD=2.7V\n57855 S1(68)=1.96LSB \\ REM ABS MAX ADC ADIN INL ERROR, VDD=4/48/80V, S+=48V\n57860 S1(69)=1.96LSB \\ REM ABS MAX ADC VIN (VDD&S+) INL ERROR, S+=48V\n57865 S1(70)=3.06LSB \\ REM ABS MAX ADC DELTA VSENSE VOS, VDD=2.7V\n57870 S1(71)=1.06LSB \\ REM ABS MAX ADC ADIN VOS, VDD=2.7V\n57875 S1(72)=1.46LSB \\ REM ABS MAX ADC VIN (VDD&S+) VOS, S+=48V\n57880 S1(73)=19.6MS  \\ REM MIN VIN/ADIN CONVERSION TIME @ VDD=S+=S-=48V\n57885 S1(74)=47.5MS  \\ REM MAX VIN/ADIN CONVERSION TIME @ VDD=S+=S-=48V\n57890 S1(75)=39.2MS  \\ REM MIN DVSEN CONVERSION TIME @ VDD=S+=S-=48V\n57895 S1(76)=95.0MS  \\ REM MAX DVSEN CONVERSION TIME @ VDD=S+=S-=48V\n57900 S1(77)=5.3HZ   \\ REM MIN CONVERSION RATE @ VDD=S+=S-=48V\n57905 S1(78)=12.8HZ  \\ REM MAX CONVERSION RATE @ VDD=S+=S-=48V\n57910 Z0=1\n57915 RETURN\n57920 SEGMENT TO MEMORY"
  # "100   K1=0    \\ REM 0=SKIP TRIM, 1=TRIM ALL\n110   MODE3=0 \\ REM 0=NOT CHAR, 1=CHAR\n120   REM MODE2=1 \\ REM 0=SKIP RE-CAL, 1=RE-CAL ALL ADC VOLTAGE OFFSETS\n130   Z=2     \\ REM 0=EHIO, 1=EWR, 2=EFR, 3=EQR, 4=EQT, 5=EQHT\n140   Y=1     \\ REM 0=LTC2945, 1=LTC2945-1"
  # "#via_ignore Spell Check\nThis is expected variable naming."
  # "Store stimulus, measurements & results"
  n1 = call "Get Class from TSM Context.vi"("TSM Context"="TSM context") -> ("Global Memory Class"=w6:refnum<class "TSM Context Data Access.lvclass">)  [unwired: 14 in]
  n2 = while {
    shift-right: [w16] -> w10
    shift-left: errorcluster {"status"=FALSE, "code"=0, "source"=""} ("error in") -> [w23]
    tunnel: "TSM context" -> [w21]
    shift-right: [w18] -> _
    shift-left: T12 {"Number Of Sites"=0, "Site Numbers"=[], "RLY12V_MEAS"={"Pin Query Context"=refnum, "SSC"=[], "Site Numbers"=[], "Pins"=[], "Pins Expanded"=[]}, "Relays Filtered Pins"=[], "Relay Pin Sessions"=[], "UDB_EN"={"Pin Query Context"=refnum, "SSC"=[], "Site Numbers"=[]}} -> [w19]
    shift-right: [w15] -> w2
    shift-left: T3 {"unloaded12VRLY"=[], "vdiode"=[], "RelayDrop"=[], "Initial Configurations"={"K1"=0, "MODE3"=0, "MODE2"=0, "Z"=0, "Y"=0}} -> [w14]
    tunnel: w6 -> [w13]
    tunnel: "TestFlowID" -> [w12]
    tunnel: "configuration file path" -> [w11]
    i -> [w24]
    stop <- w17 stop-if-true
    # "Initialise Globals"
    n3 = Increment(x=w24) -> (x+1=w22:i32)
    n4 = case shown="1" w22 {
      tunnel: [w32 w105 w171 w256 w341 w426 w511 w596 w651 w671 w681 w687] -> w16
      tunnel: w23 -> [w47 w107 w177 w262 w347 w432 w517 w602 w661 w673 w679 w687]
      tunnel: w21 -> [w46 _ _ _ _ _ _ _ _ _ _ _]
      tunnel: [_ _ _ _ _ _ _ _ _ _ _ TRUE] -> w20
      tunnel: w19 -> [w43 w110 w180 w265 w350 w435 w520 w605 w667 w675 w680 w686]
      tunnel: [w42 w110 w180 w265 w350 w435 w520 w605 w667 w675 w680 w686] -> w18
      tunnel: [w33 w109 w179 w264 w349 w434 w519 w604 w666 w674 w684 w685] -> w15
      tunnel: w14 -> [w34 w109 w179 w264 w349 w434 w519 w604 w666 w674 w684 w685]
      tunnel: w13 -> [w44 w106 w176 w261 w346 w431 w516 w601 w662 w670 w678 _]
      tunnel: w12 -> [w25 w108 w178 w263 w348 w433 w518 w603 _ _ _ _]
      tunnel: w11 -> [_ _ _ _ _ _ _ _ _ w668 _ _]
      frame 1 {
        # "#31Jan2023 Added TestFlowID global"
        # "#Debug\nThis is to transfer the config values to FileGlobals in TestStand."
        # "#TBD"
        # "Initialise Globals"
        n5 = call <vilib>:"GetSiteNumbers.vi"("error in (no error)"=w47, "Semiconductor Module Context"=w46) -> ("error out"=w45:errorcluster, "Number Of Sites"=w40:i32)  [unwired: 6 in, 2 out]
        n6 = case shown="\"LTC2945_EQR_SKIP_TRIM\"" w25 {
          tunnel: [i8 0 ("K1") i8 0 ("K1") i8 1 ("K1") i8 0 ("K1") i8 0 ("K1") i8 0 ("K1") i8 0 ("K1") i8 1 ("K1") i8 0 ("K1") i8 0 ("K1") i8 0 ("K1")] -> w39
          tunnel: [i8 1 ("K1") i8 0 ("K1") i8 0 ("K1") i8 0 ("K1") i8 0 ("K1") i8 0 ("K1") i8 0 ("K1") i8 0 ("K1") i8 0 ("K1") i8 0 ("K1") i8 0 ("K1")] -> w38
          tunnel: [i8 3 ("K1") i8 2 ("K1") i8 2 ("K1") i8 5 ("K1") i8 3 ("K1") i8 4 ("K1") i8 2 ("K1") i8 2 ("K1") i8 5 ("K1") i8 3 ("K1") i8 4 ("K1")] -> w37
          tunnel: [i8 0 ("Y") i8 0 ("Y") i8 0 ("Y") i8 0 ("Y") i8 0 ("Y") i8 0 ("Y") i8 1 ("Y") i8 1 ("Y") i8 1 ("Y") i8 1 ("Y") i8 1 ("Y")] -> w36
          frame "LTC2945_CORR_DELTA" {
          }
          frame "LTC2945_EFR_SKIP_TRIM", Default {
          }
          frame "LTC2945_EFR_TRIM_ALL" {
          }
          frame "LTC2945_EQHT_SKIP_TRIM" {
          }
          frame "LTC2945_EQR_SKIP_TRIM" {
          }
          frame "LTC2945_EQT_SKIP_TRIM" {
          }
          frame "LTC2945-1_EFR_SKIP_TRIM" {
          }
          frame "LTC2945-1_EFR_TRIM_ALL" {
          }
          frame "LTC2945-1_EQHT_SKIP_TRIM" {
          }
          frame "LTC2945-1_EQR_SKIP_TRIM" {
          }
          frame "LTC2945-1_EQT_SKIP_TRIM" {
          }
        }
        n7 = property class="Globals"(reference=w44, error in=w45, "Properties:K1"=w39, "Properties:MODE3"=w38, "Properties:Z"=w37, "Properties:Y"=w36, "Properties:MODE2"=i8 1 ("MODE2"), "Properties:TestFlowID"=w25) -> (reference out=w31:refnum<class "TSM Context Data Access.lvclass">, error out=w41:errorcluster)
        n8 = property class="Globals"(reference=w31, error in=w41) -> (error out=w32:errorcluster, "Properties:K1"=w30:i8, "Properties:MODE3"=w29:i8, "Properties:MODE2"=w28:i8, "Properties:Z"=w27:i8, "Properties:Y"=w26:i8)  [unwired: 1 out]
        n9 = Bundle By Name(cluster=w34, "Initial Configurations.K1"=w30, "Initial Configurations.MODE3"=w29, "Initial Configurations.MODE2"=w28, "Initial Configurations.Z"=w27, "Initial Configurations.Y"=w26) -> (w33:T3)
        n10 = Bundle By Name(cluster=w43, "Number Of Sites"=w40) -> (w42:T12)
      }
      frame 2 {
        # "Initialise S1(1) to S1(12)"
        # "Initialise Globals for S1 array based on TestFlowID"
        n11 = case shown="\"LTC2945_CORR_DELTA\"" w108 {
          tunnel: [w122 w134 w146 w158 w170] -> w104
          tunnel: [w121 w133 w145 w157 w169] -> w103
          tunnel: [w120 w132 w144 w156 w168] -> w102
          tunnel: [w119 w131 w143 w155 w167] -> w101
          tunnel: [w118 w130 w142 w154 w166] -> w100
          tunnel: [w117 w129 w141 w153 w165] -> w99
          tunnel: [w116 w128 w140 w152 w164] -> w98
          tunnel: [w115 w127 w139 w151 w163] -> w97
          tunnel: [w114 w126 w138 w150 w162] -> w96
          tunnel: [w113 w125 w137 w149 w161] -> w95
          tunnel: [w112 w124 w136 w148 w160] -> w94
          tunnel: [w111 w123 w135 w147 w159] -> w93
          frame "LTC2945_CORR_DELTA" {
            w111 = 1.24e-05  # S1(12)
            w112 = -1.24e-05  # S1(11)
            w113 = -5.4e-07  # S1(10)
            w114 = -4.48e-06  # S1(9)
            w115 = -1.44e-06  # S1(8)
            w116 = -9.48e-06  # S1(7)
            w117 = 1.9e-05  # S1(6)
            w118 = -1e-07  # S1(5)
            w119 = 0.000136  # S1(4)
            w120 = 1.5e-05  # S1(3)
            w121 = 0.001158  # S1(2)
            w122 = 0.000149  # S1(1)
            # "Refer EWR LIMITS"
          }
          frame "LTC2945-1_EFR_SKIP_TRIM", "LTC2945-1_EFR_TRIM_ALL", "LTC2945_EFR_SKIP_TRIM", "LTC2945_EFR_TRIM_ALL", Default {
            w123 = 1.25e-05  # S1(12)
            w124 = -1.25e-05  # S1(11)
            w125 = -4.6e-07  # S1(10)
            w126 = -4.56e-06  # S1(9)
            w127 = -1.36e-06  # S1(8)
            w128 = -9.56e-06  # S1(7)
            w129 = 1.92e-05  # S1(6)
            w130 = -3e-07  # S1(5)
            w131 = 0.000138  # S1(4)
            w132 = 1.3e-05  # S1(3)
            w133 = 0.001161  # S1(2)
            w134 = 0.000146  # S1(1)
            # "Refer EFR LIMITS"
          }
          frame "LTC2945-1_EQR_SKIP_TRIM", "LTC2945_EQR_SKIP_TRIM" {
            w135 = 1.28e-05  # S1(12)
            w136 = -1.28e-05  # S1(11)
            w137 = -8e-08  # S1(10)
            w138 = -4.84e-06  # S1(9)
            w139 = -1.08e-06  # S1(8)
            w140 = -9.84e-06  # S1(7)
            w141 = 1.96e-05  # S1(6)
            w142 = -8e-07  # S1(5)
            w143 = 0.000146  # S1(4)
            w144 = 3e-06  # S1(3)
            w145 = 0.001194  # S1(2)
            w146 = 0.000103  # S1(1)
            # "Refer EQR LIMITS"
          }
          frame "LTC2945-1_EQT_SKIP_TRIM", "LTC2945_EQT_SKIP_TRIM" {
            w147 = 1.29e-05  # S1(12)
            w148 = -1.29e-05  # S1(11)
            w149 = 0.0  # S1(10)
            w150 = -4.92e-06  # S1(9)
            w151 = -1e-06  # S1(8)
            w152 = -9.92e-06  # S1(7)
            w153 = 1.98e-05  # S1(6)
            w154 = -1e-06  # S1(5)
            w155 = 0.000148  # S1(4)
            w156 = 1e-06  # S1(3)
            w157 = 1.197  # S1(2)
            w158 = 0.0001  # S1(1)
            # "Refer EQT LIMITS"
          }
          frame "LTC2945-1_EQHT_SKIP_TRIM", "LTC2945_EQHT_SKIP_TRIM" {
            w159 = 1.29e-05  # S1(12)
            w160 = -1.29e-05  # S1(11)
            w161 = 0.0  # S1(10)
            w162 = -4.92e-06  # S1(9)
            w163 = -1e-06  # S1(8)
            w164 = -9.92e-06  # S1(7)
            w165 = 1.98e-05  # S1(6)
            w166 = -1e-06  # S1(5)
            w167 = 0.000148  # S1(4)
            w168 = 1e-06  # S1(3)
            w169 = 1.197  # S1(2)
            w170 = 0.0001  # S1(1)
            # "Refer EQHT LIMITS"
          }
        }
        n12 = Build Array(w104, w103, w102, w101, w100, w99, w98, w97, w96, w95, w94, w93) -> (w92:dbl[])
        n13 = property class="Globals"(reference=w106, error in=w107, "Properties:S1"=w92) -> (error out=w105:errorcluster)  [unwired: 1 out]
      }
      frame 3 {
        # "Initialise S1(13) to S1(24)"
        # "Initialise Globals for S1 array based on TestFlowID"
        n14 = property class="Globals"(reference=w176, error in=w177) -> (reference out=w172:refnum<class "TSM Context Data Access.lvclass">, error out=w175:errorcluster, "Properties:S1"=w174:dbl[])
        n15 = case shown="\"LTC2945-1_EFR_SKIP_TRIM\", \"LTC2945-1_EFR_TRIM_ALL\", \"LTC2945_EFR_SKIP_TRIM\", \"LTC2945_EFR_TRIM_ALL\", Default" w178 {
          tunnel: w174 -> [w194 w198 w212 w227 w242]
          tunnel: [w182 w197 w211 w226 w241] -> w173
          frame "LTC2945_CORR_DELTA" {
            w183 = 7.1e-07  # S1(24)
            w184 = -7.1e-07  # S1(23)
            w185 = 6.848  # S1(22)
            w186 = 5.912  # S1(21)
            w187 = 7.1e-07  # S1(20)
            w188 = -7.1e-07  # S1(19)
            w189 = 0.006  # S1(18)
            w190 = 0.004  # S1(17)
            w191 = 4200000.0  # S1(16)
            w192 = 7.1e-07  # S1(15)
            w193 = 1.24e-05  # S1(14)
            w195 = -1.24e-05  # S1(13)
            # "Refer EWR LIMITS"
            n16 = Insert Into Array(array=w194, index=12, new element #1=w195, new element #2=w193, new element #3=w192, new element #4=w191, new element #5=w190, new element #6=w189, new element #7=w188, new element #8=w187, new element #9=w186, new element #10=w185, new element #11=w184, new element #12=w183) -> (w182:dbl[])
          }
          frame "LTC2945-1_EFR_SKIP_TRIM", "LTC2945-1_EFR_TRIM_ALL", "LTC2945_EFR_SKIP_TRIM", "LTC2945_EFR_TRIM_ALL", Default {
            w200 = 7.8e-07  # S1(24)
            w201 = -7.8e-07  # S1(23)
            w202 = 6.851  # S1(22)
            w196 = 5.909  # S1(21)
            w203 = 7.8e-07  # S1(20)
            w204 = -7.8e-07  # S1(19)
            w205 = 0.006  # S1(18)
            w206 = 0.004  # S1(17)
            w207 = 4000000.0  # S1(16)
            w208 = 7.8e-07  # S1(15)
            w209 = 1.25e-05  # S1(14)
            w210 = -1.25e-05  # S1(13)
            # "Refer EFR LIMITS"
            n17 = Insert Into Array(array=w198, index=12, new element #1=w210, new element #2=w209, new element #3=w208, new element #4=w207, new element #5=w206, new element #6=w205, new element #7=w204, new element #8=w203, new element #9=w196, new element #10=w202, new element #11=w201, new element #12=w200) -> (w197:dbl[])
          }
          frame "LTC2945-1_EQR_SKIP_TRIM", "LTC2945_EQR_SKIP_TRIM" {
            w215 = 8.6e-07  # S1(24)
            w216 = -8.6e-07  # S1(23)
            w217 = 6.894  # S1(22)
            w213 = 5.906  # S1(21)
            w218 = 8.6e-07  # S1(20)
            w219 = -8.6e-07  # S1(19)
            w220 = 0.009  # S1(18)
            w221 = 0.006  # S1(17)
            w222 = 3400000.0  # S1(16)
            w223 = 8.6e-07  # S1(15)
            w224 = 1.28e-05  # S1(14)
            w225 = -1.28e-05  # S1(13)
            # "Refer EQR LIMITS"
            n18 = Insert Into Array(array=w212, index=12, new element #1=w225, new element #2=w224, new element #3=w223, new element #4=w222, new element #5=w221, new element #6=w220, new element #7=w219, new element #8=w218, new element #9=w213, new element #10=w217, new element #11=w216, new element #12=w215) -> (w211:dbl[])
          }
          frame "LTC2945-1_EQT_SKIP_TRIM", "LTC2945_EQT_SKIP_TRIM" {
            w230 = 9.3e-07  # S1(24)
            w231 = -9.3e-07  # S1(23)
            w232 = 6.897  # S1(22)
            w228 = 5.903  # S1(21)
            w233 = 9.3e-07  # S1(20)
            w234 = -9.3e-07  # S1(19)
            w235 = 0.012  # S1(18)
            w236 = 0.008  # S1(17)
            w237 = 3200000.0  # S1(16)
            w238 = 9.3e-07  # S1(15)
            w239 = 1.29e-05  # S1(14)
            w240 = -1.29e-05  # S1(13)
            # "Refer EQT LIMITS"
            n19 = Insert Into Array(array=w227, index=12, new element #1=w240, new element #2=w239, new element #3=w238, new element #4=w237, new element #5=w236, new element #6=w235, new element #7=w234, new element #8=w233, new element #9=w228, new element #10=w232, new element #11=w231, new element #12=w230) -> (w226:dbl[])
          }
          frame "LTC2945-1_EQHT_SKIP_TRIM", "LTC2945_EQHT_SKIP_TRIM" {
            w245 = 9.3e-07  # S1(24)
            w246 = -9.3e-07  # S1(23)
            w247 = 6.897  # S1(22)
            w243 = 5.903  # S1(21)
            w248 = 9.3e-07  # S1(20)
            w249 = -9.3e-07  # S1(19)
            w250 = 0.012  # S1(18)
            w251 = 0.008  # S1(17)
            w252 = 3200000.0  # S1(16)
            w253 = 9.3e-07  # S1(15)
            w254 = 1.29e-05  # S1(14)
            w255 = -1.29e-05  # S1(13)
            # "Refer EQHT LIMITS"
            n20 = Insert Into Array(array=w242, index=12, new element #1=w255, new element #2=w254, new element #3=w253, new element #4=w252, new element #5=w251, new element #6=w250, new element #7=w249, new element #8=w248, new element #9=w243, new element #10=w247, new element #11=w246, new element #12=w245) -> (w241:dbl[])
          }
        }
        n21 = property class="Globals"(reference=w172, error in=w175, "Properties:S1"=w173) -> (error out=w171:errorcluster)  [unwired: 1 out]
      }
      frame 4 {
        # "Initialise S1(25) to S1(36)"
        # "Initialise Globals for S1 array based on TestFlowID"
        n22 = property class="Globals"(reference=w261, error in=w262) -> (reference out=w257:refnum<class "TSM Context Data Access.lvclass">, error out=w260:errorcluster, "Properties:S1"=w259:dbl[])
        n23 = case shown="\"LTC2945-1_EQHT_SKIP_TRIM\", \"LTC2945_EQHT_SKIP_TRIM\"" w263 {
          tunnel: w259 -> [w279 w283 w297 w312 w327]
          tunnel: [w267 w282 w296 w311 w326] -> w258
          frame "LTC2945_CORR_DELTA" {
            w268 = 6.3e-05  # S1(36)
            w269 = 3.5e-05  # S1(35)
            w270 = 7.9e-07  # S1(34)
            w271 = 1.7e-06  # S1(33)
            w272 = 0.18  # S1(32)
            w273 = 5.258  # S1(31)
            w274 = 4.772  # S1(30)
            w275 = 0.213  # S1(29)
            w276 = 6.638  # S1(28)
            w277 = 5.932  # S1(27)
            w278 = 0.000862  # S1(26)
            w280 = 5.6e-05  # S1(25)
            # "Refer EWR LIMITS"
            n24 = Insert Into Array(array=w279, index=24, new element #1=w280, new element #2=w278, new element #3=w277, new element #4=w276, new element #5=w275, new element #6=w274, new element #7=w273, new element #8=w272, new element #9=w271, new element #10=w270, new element #11=w269, new element #12=w268) -> (w267:dbl[])
          }
          frame "LTC2945-1_EFR_SKIP_TRIM", "LTC2945-1_EFR_TRIM_ALL", "LTC2945_EFR_SKIP_TRIM", "LTC2945_EFR_TRIM_ALL", Default {
            w281 = 6.4e-05  # S1(36)
            w285 = 3.7e-05  # S1(35)
            w286 = 8.3e-07  # S1(34)
            w287 = 1.74e-06  # S1(33)
            w288 = 0.182  # S1(32)
            w289 = 5.261  # S1(31)
            w290 = 4.769  # S1(30)
            w291 = 0.216  # S1(29)
            w292 = 6.641  # S1(28)
            w293 = 5.929  # S1(27)
            w294 = 0.000864  # S1(26)
            w295 = 5.4e-05  # S1(25)
            # "Refer EFR LIMITS"
            # "Refer EFR LIMITS"
            n25 = Insert Into Array(array=w283, index=24, new element #1=w295, new element #2=w294, new element #3=w293, new element #4=w292, new element #5=w291, new element #6=w290, new element #7=w289, new element #8=w288, new element #9=w287, new element #10=w286, new element #11=w285, new element #12=w281) -> (w282:dbl[])
          }
          frame "LTC2945-1_EQR_SKIP_TRIM", "LTC2945_EQR_SKIP_TRIM" {
            w298 = 6.7e-05  # S1(36)
            w300 = 7.7e-05  # S1(35)
            w301 = 8.8e-07  # S1(34)
            w302 = 1.88e-06  # S1(33)
            w303 = 0.196  # S1(32)
            w304 = 5.494  # S1(31)
            w305 = 4.506  # S1(30)
            w306 = 0.244  # S1(29)
            w307 = 6.694  # S1(28)
            w308 = 5.906  # S1(27)
            w309 = 0.000896  # S1(26)
            w310 = 1.2e-05  # S1(25)
            # "Refer EQR LIMITS"
            n26 = Insert Into Array(array=w297, index=24, new element #1=w310, new element #2=w309, new element #3=w308, new element #4=w307, new element #5=w306, new element #6=w305, new element #7=w304, new element #8=w303, new element #9=w302, new element #10=w301, new element #11=w300, new element #12=w298) -> (w296:dbl[])
          }
          frame "LTC2945-1_EQT_SKIP_TRIM", "LTC2945_EQT_SKIP_TRIM" {
            w313 = 6.9e-05  # S1(36)
            w315 = 7.9e-05  # S1(35)
            w316 = 9.2e-07  # S1(34)
            w317 = 1.92e-06  # S1(33)
            w318 = 0.198  # S1(32)
            w319 = 5.497  # S1(31)
            w320 = 4.503  # S1(30)
            w321 = 0.247  # S1(29)
            w322 = 6.697  # S1(28)
            w323 = 5.903  # S1(27)
            w324 = 0.000898  # S1(26)
            w325 = 1e-05  # S1(25)
            # "Refer EQT LIMITS"
            n27 = Insert Into Array(array=w312, index=24, new element #1=w325, new element #2=w324, new element #3=w323, new element #4=w322, new element #5=w321, new element #6=w320, new element #7=w319, new element #8=w318, new element #9=w317, new element #10=w316, new element #11=w315, new element #12=w313) -> (w311:dbl[])
          }
          frame "LTC2945-1_EQHT_SKIP_TRIM", "LTC2945_EQHT_SKIP_TRIM" {
            w328 = 6.9e-05  # S1(36)
            w330 = 7.9e-05  # S1(35)
            w331 = 9.2e-07  # S1(34)
            w332 = 1.92e-06  # S1(33)
            w333 = 0.198  # S1(32)
            w334 = 5.697  # S1(31)
            w335 = 4.503  # S1(30)
            w336 = 0.247  # S1(29)
            w337 = 6.697  # S1(28)
            w338 = 5.903  # S1(27)
            w339 = 0.000898  # S1(26)
            w340 = 1e-05  # S1(25)
            # "Refer EQHT LIMITS"
            n28 = Insert Into Array(array=w327, index=24, new element #1=w340, new element #2=w339, new element #3=w338, new element #4=w337, new element #5=w336, new element #6=w335, new element #7=w334, new element #8=w333, new element #9=w332, new element #10=w331, new element #11=w330, new element #12=w328) -> (w326:dbl[])
          }
        }
        n29 = property class="Globals"(reference=w257, error in=w260, "Properties:S1"=w258) -> (error out=w256:errorcluster)  [unwired: 1 out]
      }
      frame 5 {
        # "Initialise S1(37) to S1(48)"
        # "Initialise Globals for S1 array based on TestFlowID"
        n30 = property class="Globals"(reference=w346, error in=w347) -> (reference out=w342:refnum<class "TSM Context Data Access.lvclass">, error out=w345:errorcluster, "Properties:S1"=w344:dbl[])
        n31 = case shown="\"LTC2945-1_EQHT_SKIP_TRIM\", \"LTC2945_EQHT_SKIP_TRIM\"" w348 {
          tunnel: w344 -> [w364 w367 w382 w397 w413]
          tunnel: [w352 w366 w381 w396 w412] -> w343
          frame "LTC2945_CORR_DELTA" {
            w353 = 2.35  # S1(48)
            w354 = 2.11  # S1(47)
            w355 = 1.59  # S1(46)
            w356 = 0.322  # S1(45)
            w357 = 0.086  # S1(44)
            w358 = 0.8  # S1(43)
            w359 = 0.4  # S1(42)
            w360 = 2.6  # S1(41)
            w361 = 2.0  # S1(40)
            w362 = 0.52  # S1(39)
            w363 = 0.52  # S1(38)
            w365 = 0.52  # S1(37)
            # "Refer EWR LIMITS"
            n32 = Insert Into Array(array=w364, index=36, new element #1=w365, new element #2=w363, new element #3=w362, new element #4=w361, new element #5=w360, new element #6=w359, new element #7=w358, new element #8=w357, new element #9=w356, new element #10=w355, new element #11=w354, new element #12=w353) -> (w352:dbl[])
          }
          frame "LTC2945-1_EFR_SKIP_TRIM", "LTC2945-1_EFR_TRIM_ALL", "LTC2945_EFR_SKIP_TRIM", "LTC2945_EFR_TRIM_ALL", Default {
            w369 = 2.34  # S1(48)
            w370 = 2.13  # S1(47)
            w371 = 1.57  # S1(46)
            w372 = 0.324  # S1(45)
            w373 = 0.084  # S1(44)
            w374 = 0.82  # S1(43)
            w375 = 0.38  # S1(42)
            w376 = 2.62  # S1(41)
            w377 = 1.98  # S1(40)
            w378 = 0.54  # S1(39)
            w379 = 0.54  # S1(38)
            w380 = 0.54  # S1(37)
            # "Refer EFR LIMITS"
            # "Refer EFR LIMITS"
            n33 = Insert Into Array(array=w367, index=36, new element #1=w380, new element #2=w379, new element #3=w378, new element #4=w377, new element #5=w376, new element #6=w375, new element #7=w374, new element #8=w373, new element #9=w372, new element #10=w371, new element #11=w370, new element #12=w369) -> (w366:dbl[])
          }
          frame "LTC2945-1_EQR_SKIP_TRIM", "LTC2945_EQR_SKIP_TRIM" {
            w384 = 2.32  # S1(48)
            w385 = 2.16  # S1(47)
            w386 = 1.54  # S1(46)
            w387 = 0.396  # S1(45)
            w388 = 0.012  # S1(44)
            w389 = 0.86  # S1(43)
            w390 = 0.34  # S1(42)
            w391 = 2.66  # S1(41)
            w392 = 1.94  # S1(40)
            w393 = 0.71  # S1(39)
            w394 = 0.71  # S1(38)
            w395 = 0.71  # S1(37)
            # "Refer EQR LIMITS"
            n34 = Insert Into Array(array=w382, index=36, new element #1=w395, new element #2=w394, new element #3=w393, new element #4=w392, new element #5=w391, new element #6=w390, new element #7=w389, new element #8=w388, new element #9=w387, new element #10=w386, new element #11=w385, new element #12=w384) -> (w381:dbl[])
          }
          frame "LTC2945-1_EQT_SKIP_TRIM", "LTC2945_EQT_SKIP_TRIM" {
            w399 = 2.31  # S1(48)
            w400 = 2.18  # S1(47)
            w401 = 1.52  # S1(46)
            w402 = 0.398  # S1(45)
            w403 = 0.01  # S1(44)
            w404 = 0.88  # S1(43)
            w405 = 0.32  # S1(42)
            w406 = 2.68  # S1(41)
            w407 = 1.92  # S1(40)
            w408 = 0.73  # S1(39)
            w409 = 0.73  # S1(38)
            w410 = 0.73  # S1(37)
            # "Refer EQT LIMITS"
            n35 = Insert Into Array(array=w397, index=36, new element #1=w410, new element #2=w409, new element #3=w408, new element #4=w407, new element #5=w406, new element #6=w405, new element #7=w404, new element #8=w403, new element #9=w402, new element #10=w401, new element #11=w400, new element #12=w399) -> (w396:dbl[])
          }
          frame "LTC2945-1_EQHT_SKIP_TRIM", "LTC2945_EQHT_SKIP_TRIM" {
            w411 = 2.31  # S1(48)
            w415 = 2.18  # S1(47)
            w416 = 1.52  # S1(46)
            w417 = 0.398  # S1(45)
            w418 = 0.01  # S1(44)
            w419 = 0.88  # S1(43)
            w420 = 0.32  # S1(42)
            w421 = 2.68  # S1(41)
            w422 = 1.92  # S1(40)
            w423 = 0.73  # S1(39)
            w424 = 0.73  # S1(38)
            w425 = 0.73  # S1(37)
            # "Refer EQHT LIMITS"
            n36 = Insert Into Array(array=w413, index=36, new element #1=w425, new element #2=w424, new element #3=w423, new element #4=w422, new element #5=w421, new element #6=w420, new element #7=w419, new element #8=w418, new element #9=w417, new element #10=w416, new element #11=w415, new element #12=w411) -> (w412:dbl[])
          }
        }
        n37 = property class="Globals"(reference=w342, error in=w345, "Properties:S1"=w343) -> (error out=w341:errorcluster)  [unwired: 1 out]
      }
      frame 6 {
        # "Initialise S1(49) to S1(60)"
        # "Initialise Globals for S1 array based on TestFlowID"
        n38 = property class="Globals"(reference=w431, error in=w432) -> (reference out=w427:refnum<class "TSM Context Data Access.lvclass">, error out=w430:errorcluster, "Properties:S1"=w429:dbl[])
        n39 = case shown="\"LTC2945-1_EQHT_SKIP_TRIM\", \"LTC2945_EQHT_SKIP_TRIM\"" w433 {
          tunnel: w429 -> [w437 w452 w467 w482 w497]
          tunnel: [w436 w451 w466 w481 w496] -> w428
          frame "LTC2945_CORR_DELTA" {
            w438 = 0.05  # S1(60)
            w440 = 0.025  # S1(59)
            w441 = 0.0  # S1(58)
            w442 = 0.0  # S1(57)
            w443 = 0.0  # S1(56)
            w444 = 3.02  # S1(55)
            w445 = 2.19  # S1(54)
            w446 = 2.45  # S1(53)
            w447 = 1.66  # S1(52)
            w448 = 3.3  # S1(51)
            w449 = 3.08  # S1(50)
            w450 = 2.64  # S1(49)
            # "Refer EWR LIMITS"
            n40 = Insert Into Array(array=w437, index=48, new element #1=w450, new element #2=w449, new element #3=w448, new element #4=w447, new element #5=w446, new element #6=w445, new element #7=w444, new element #8=w443, new element #9=w442, new element #10=w441, new element #11=w440, new element #12=w438) -> (w436:dbl[])
          }
          frame "LTC2945-1_EFR_SKIP_TRIM", "LTC2945-1_EFR_TRIM_ALL", "LTC2945_EFR_SKIP_TRIM", "LTC2945_EFR_TRIM_ALL", Default {
            w453 = 0.05  # S1(60)
            w455 = 0.025  # S1(59)
            w456 = 0.0  # S1(58)
            w457 = 0.0  # S1(57)
            w458 = 0.0  # S1(56)
            w459 = 3.03  # S1(55)
            w460 = 2.18  # S1(54)
            w461 = 2.46  # S1(53)
            w462 = 1.65  # S1(52)
            w463 = 3.32  # S1(51)
            w464 = 3.06  # S1(50)
            w465 = 2.65  # S1(49)
            # "Refer EFR LIMITS"
            # "Refer EFR LIMITS"
            n41 = Insert Into Array(array=w452, index=48, new element #1=w465, new element #2=w464, new element #3=w463, new element #4=w462, new element #5=w461, new element #6=w460, new element #7=w459, new element #8=w458, new element #9=w457, new element #10=w456, new element #11=w455, new element #12=w453) -> (w451:dbl[])
          }
          frame "LTC2945-1_EQR_SKIP_TRIM", "LTC2945_EQR_SKIP_TRIM" {
            w468 = 0.05  # S1(60)
            w470 = 0.025  # S1(59)
            w471 = 0.0  # S1(58)
            w472 = 0.0  # S1(57)
            w473 = 0.0  # S1(56)
            w474 = 3.19  # S1(55)
            w475 = 2.02  # S1(54)
            w476 = 2.59  # S1(53)
            w477 = 1.52  # S1(52)
            w478 = 3.46  # S1(51)
            w479 = 2.94  # S1(50)
            w480 = 2.67  # S1(49)
            # "Refer EQR LIMITS"
            n42 = Insert Into Array(array=w467, index=48, new element #1=w480, new element #2=w479, new element #3=w478, new element #4=w477, new element #5=w476, new element #6=w475, new element #7=w474, new element #8=w473, new element #9=w472, new element #10=w471, new element #11=w470, new element #12=w468) -> (w466:dbl[])
          }
          frame "LTC2945-1_EQT_SKIP_TRIM", "LTC2945_EQT_SKIP_TRIM" {
            w483 = 0.05  # S1(60)
            w485 = 0.025  # S1(59)
            w486 = 0.0  # S1(58)
            w487 = 0.0  # S1(57)
            w488 = 0.0  # S1(56)
            w489 = 3.2  # S1(55)
            w490 = 2.01  # S1(54)
            w491 = 2.6  # S1(53)
            w492 = 1.51  # S1(52)
            w493 = 3.48  # S1(51)
            w494 = 2.92  # S1(50)
            w495 = 2.68  # S1(49)
            # "Refer EQT LIMITS"
            n43 = Insert Into Array(array=w482, index=48, new element #1=w495, new element #2=w494, new element #3=w493, new element #4=w492, new element #5=w491, new element #6=w490, new element #7=w489, new element #8=w488, new element #9=w487, new element #10=w486, new element #11=w485, new element #12=w483) -> (w481:dbl[])
          }
          frame "LTC2945-1_EQHT_SKIP_TRIM", "LTC2945_EQHT_SKIP_TRIM" {
            w498 = 0.05  # S1(60)
            w500 = 0.025  # S1(59)
            w501 = 0.0  # S1(58)
            w502 = 0.0  # S1(57)
            w503 = 0.0  # S1(56)
            w504 = 3.2  # S1(55)
            w505 = 1.71  # S1(54)
            w506 = 2.6  # S1(53)
            w507 = 1.51  # S1(52)
            w508 = 3.48  # S1(51)
            w509 = 2.62  # S1(50)
            w510 = 2.68  # S1(49)
            # "Refer EQHT LIMITS"
            n44 = Insert Into Array(array=w497, index=48, new element #1=w510, new element #2=w509, new element #3=w508, new element #4=w507, new element #5=w506, new element #6=w505, new element #7=w504, new element #8=w503, new element #9=w502, new element #10=w501, new element #11=w500, new element #12=w498) -> (w496:dbl[])
          }
        }
        n45 = property class="Globals"(reference=w427, error in=w430, "Properties:S1"=w428) -> (error out=w426:errorcluster)  [unwired: 1 out]
      }
      frame 7 {
        # "Initialise S1(61) to S1(72)"
        # "Initialise Globals for S1 array based on TestFlowID"
        n46 = property class="Globals"(reference=w516, error in=w517) -> (reference out=w512:refnum<class "TSM Context Data Access.lvclass">, error out=w515:errorcluster, "Properties:S1"=w514:dbl[])
        n47 = case shown="\"LTC2945-1_EQHT_SKIP_TRIM\", \"LTC2945_EQHT_SKIP_TRIM\"" w518 {
          tunnel: w514 -> [w522 w537 w552 w567 w582]
          tunnel: [w521 w536 w551 w566 w581] -> w513
          frame "LTC2945_CORR_DELTA" {
            w523 = 1.46  # S1(72)
            w525 = 1.06  # S1(71)
            w526 = 3.06  # S1(70)
            w527 = 1.96  # S1(69)
            w528 = 1.96  # S1(68)
            w529 = 2.96  # S1(67)
            w530 = 3.92e-05  # S1(66)
            w531 = 6e-07  # S1(65)
            w532 = 0.000188  # S1(64)
            w533 = 1.5e-05  # S1(63)
            w534 = 0.00195  # S1(62)
            w535 = 0.00027  # S1(61)
            # "Refer EWR LIMITS"
            n48 = Insert Into Array(array=w522, index=60, new element #1=w535, new element #2=w534, new element #3=w533, new element #4=w532, new element #5=w531, new element #6=w530, new element #7=w529, new element #8=w528, new element #9=w527, new element #10=w526, new element #11=w525, new element #12=w523) -> (w521:dbl[])
          }
          frame "LTC2945-1_EFR_SKIP_TRIM", "LTC2945-1_EFR_TRIM_ALL", "LTC2945_EFR_SKIP_TRIM", "LTC2945_EFR_TRIM_ALL", Default {
            w538 = 1.47  # S1(72)
            w540 = 1.07  # S1(71)
            w541 = 3.07  # S1(70)
            w542 = 1.97  # S1(69)
            w543 = 1.97  # S1(68)
            w544 = 2.97  # S1(67)
            w545 = 3.94e-05  # S1(66)
            w546 = 4e-07  # S1(65)
            w547 = 0.00019  # S1(64)
            w548 = 1.3e-05  # S1(63)
            w549 = 0.00196  # S1(62)
            w550 = 0.00026  # S1(61)
            # "Refer EFR LIMITS"
            # "Refer EFR LIMITS"
            n49 = Insert Into Array(array=w537, index=60, new element #1=w550, new element #2=w549, new element #3=w548, new element #4=w547, new element #5=w546, new element #6=w545, new element #7=w544, new element #8=w543, new element #9=w542, new element #10=w541, new element #11=w540, new element #12=w538) -> (w536:dbl[])
          }
          frame "LTC2945-1_EQR_SKIP_TRIM", "LTC2945_EQR_SKIP_TRIM" {
            w553 = 1.48  # S1(72)
            w555 = 1.08  # S1(71)
            w556 = 3.08  # S1(70)
            w557 = 1.98  # S1(69)
            w558 = 1.98  # S1(68)
            w559 = 2.98  # S1(67)
            w560 = 3.98e-05  # S1(66)
            w561 = 0.0  # S1(65)
            w562 = 0.000198  # S1(64)
            w563 = 3e-06  # S1(63)
            w564 = 0.00199  # S1(62)
            w565 = 0.00021  # S1(61)
            # "Refer EQR LIMITS"
            n50 = Insert Into Array(array=w552, index=60, new element #1=w565, new element #2=w564, new element #3=w563, new element #4=w562, new element #5=w561, new element #6=w560, new element #7=w559, new element #8=w558, new element #9=w557, new element #10=w556, new element #11=w555, new element #12=w553) -> (w551:dbl[])
          }
          frame "LTC2945-1_EQT_SKIP_TRIM", "LTC2945_EQT_SKIP_TRIM" {
            w568 = 1.49  # S1(72)
            w570 = 1.09  # S1(71)
            w571 = 3.09  # S1(70)
            w572 = 1.99  # S1(69)
            w573 = 1.99  # S1(68)
            w574 = 2.99  # S1(67)
            w575 = 4e-05  # S1(66)
            w576 = -2e-07  # S1(65)
            w577 = 0.0002  # S1(64)
            w578 = 1e-06  # S1(63)
            w579 = 0.002  # S1(62)
            w580 = 0.0002  # S1(61)
            # "Refer EQT LIMITS"
            n51 = Insert Into Array(array=w567, index=60, new element #1=w580, new element #2=w579, new element #3=w578, new element #4=w577, new element #5=w576, new element #6=w575, new element #7=w574, new element #8=w573, new element #9=w572, new element #10=w571, new element #11=w570, new element #12=w568) -> (w566:dbl[])
          }
          frame "LTC2945-1_EQHT_SKIP_TRIM", "LTC2945_EQHT_SKIP_TRIM" {
            w583 = 1.49  # S1(72)
            w585 = 1.09  # S1(71)
            w586 = 3.09  # S1(70)
            w587 = 1.99  # S1(69)
            w588 = 1.99  # S1(68)
            w589 = 2.99  # S1(67)
            w590 = 4e-05  # S1(66)
            w591 = -2e-07  # S1(65)
            w592 = 0.0002  # S1(64)
            w593 = 1e-06  # S1(63)
            w594 = 0.002  # S1(62)
            w595 = 0.0002  # S1(61)
            # "Refer EQHT LIMITS"
            n52 = Insert Into Array(array=w582, index=60, new element #1=w595, new element #2=w594, new element #3=w593, new element #4=w592, new element #5=w591, new element #6=w590, new element #7=w589, new element #8=w588, new element #9=w587, new element #10=w586, new element #11=w585, new element #12=w583) -> (w581:dbl[])
          }
        }
        n53 = property class="Globals"(reference=w512, error in=w515, "Properties:S1"=w513) -> (error out=w511:errorcluster)  [unwired: 1 out]
      }
      frame 8 {
        # "Initialise S1(73) to S1(78)"
        # "Initialise Globals for S1 array based on TestFlowID"
        n54 = property class="Globals"(reference=w601, error in=w602) -> (reference out=w597:refnum<class "TSM Context Data Access.lvclass">, error out=w600:errorcluster, "Properties:S1"=w599:dbl[])
        n55 = case shown="\"LTC2945-1_EQHT_SKIP_TRIM\", \"LTC2945_EQHT_SKIP_TRIM\"" w603 {
          tunnel: w599 -> [w607 w616 w625 w634 w643]
          tunnel: [w606 w615 w624 w633 w642] -> w598
          frame "LTC2945_CORR_DELTA" {
            w609 = 12.8  # S1(78)
            w610 = 5.3  # S1(77)
            w611 = 0.095  # S1(76)
            w612 = 0.0392  # S1(75)
            w613 = 0.0475  # S1(74)
            w614 = 0.0196  # S1(73)
            # "Refer EWR LIMITS"
            n56 = Insert Into Array(array=w607, index=72, new element #1=w614, new element #2=w613, new element #3=w612, new element #4=w611, new element #5=w610, new element #6=w609) -> (w606:dbl[])
          }
          frame "LTC2945-1_EFR_SKIP_TRIM", "LTC2945-1_EFR_TRIM_ALL", "LTC2945_EFR_SKIP_TRIM", "LTC2945_EFR_TRIM_ALL", Default {
            w618 = 8.95  # S1(78)
            w619 = 6.05  # S1(77)
            w620 = 0.07184  # S1(76)
            w621 = 0.0601  # S1(75)
            w622 = 0.03591  # S1(74)
            w623 = 0.03005  # S1(73)
            # "Refer EFR LIMITS"
            # "Refer EFR LIMITS"
            n57 = Insert Into Array(array=w616, index=72, new element #1=w623, new element #2=w622, new element #3=w621, new element #4=w620, new element #5=w619, new element #6=w618) -> (w615:dbl[])
          }
          frame "LTC2945-1_EQR_SKIP_TRIM", "LTC2945_EQR_SKIP_TRIM" {
            w627 = 8.98  # S1(78)
            w628 = 6.02  # S1(77)
            w629 = 0.07196  # S1(76)
            w630 = 0.06004  # S1(75)
            w631 = 0.03598  # S1(74)
            w632 = 0.03002  # S1(73)
            # "Refer EQR LIMITS"
            n58 = Insert Into Array(array=w625, index=72, new element #1=w632, new element #2=w631, new element #3=w630, new element #4=w629, new element #5=w628, new element #6=w627) -> (w624:dbl[])
          }
          frame "LTC2945-1_EQT_SKIP_TRIM", "LTC2945_EQT_SKIP_TRIM" {
            w636 = 8.99  # S1(78)
            w637 = 6.01  # S1(77)
            w638 = 0.07198  # S1(76)
            w639 = 0.06002  # S1(75)
            w640 = 0.03599  # S1(74)
            w641 = 0.03001  # S1(73)
            # "Refer EQT LIMITS"
            n59 = Insert Into Array(array=w634, index=72, new element #1=w641, new element #2=w640, new element #3=w639, new element #4=w638, new element #5=w637, new element #6=w636) -> (w633:dbl[])
          }
          frame "LTC2945-1_EQHT_SKIP_TRIM", "LTC2945_EQHT_SKIP_TRIM" {
            w645 = 8.99  # S1(78)
            w646 = 6.01  # S1(77)
            w647 = 0.07198  # S1(76)
            w648 = 0.06002  # S1(75)
            w649 = 0.03599  # S1(74)
            w650 = 0.03001  # S1(73)
            # "Refer EQHT LIMITS"
            n60 = Insert Into Array(array=w643, index=72, new element #1=w650, new element #2=w649, new element #3=w648, new element #4=w647, new element #5=w646, new element #6=w645) -> (w642:dbl[])
          }
        }
        n61 = property class="Globals"(reference=w597, error in=w600, "Properties:S1"=w598) -> (error out=w596:errorcluster)  [unwired: 1 out]
      }
      frame 9 {
        w652 = 0 ("Z1")
        w655 = 0 ("DNUM")
        # "DIM S1(250)\nHence, for rest of the index from S1(79) to S1(250) will be initialise to 0"
        # "Initialise Globals for S1 array to 0 for S1(79)-S1(250)"
        n62 = property class="Globals"(reference=w662, error in=w661) -> (reference out=w659:refnum<class "TSM Context Data Access.lvclass">, error out=w660:errorcluster, "Properties:S1"=w658:dbl[])
        n63 = Initialize Array(0.0 ("element"), 173 ("dimension size")) -> (w657:dbl[])
        n64 = Insert Into Array(array=w658, index=78, new element=w657) -> (w656:dbl[])
        n65 = property class="Globals"(reference=w659, error in=w660, "Properties:S1"=w656, "Properties:DNUM"=w655, "Properties:U0"=w655, "Properties:U1"=w655, "Properties:U2"=w655, "Properties:U3"=w655, "Properties:U4"=w655, "Properties:U5"=w655, "Properties:U7"=w655, "Properties:U8"=w655, "Properties:U9"=w655) -> (reference out=w653:refnum<class "TSM Context Data Access.lvclass">, error out=w654:errorcluster)
        n66 = property class="Globals"(reference=w653, error in=w654, "Properties:Z1"=w652, "Properties:Z2"=w652, "Properties:Z3"=w652, "Properties:Z4"=w652, "Properties:Z5"=w652, "Properties:Z6"=w652, "Properties:Z7"=w652, "Properties:Z8"=w652, "Properties:Z9"=w652) -> (error out=w651:errorcluster)  [unwired: 1 out]
      }
      frame 10 {
        # "Get Reference Data from Ini File"
        n67 = call "GetRefDatafromINIFile.vi"("error in (no error)"=w673, "RefDataIn"=w668) -> ("error out"=w672:errorcluster, "Reference Data"=w669:dbl[][])  [unwired: 7 in, 1 out]
        n68 = property class="Globals"(reference=w670, error in=w672, "Properties:ReferenceData"=w669) -> (error out=w671:errorcluster)  [unwired: 1 out]
      }
      frame 11 {
        # "Initialize Calibration Globals"
        n69 = Unbundle By Name(w680) -> ("Number Of Sites"=w677:i32)
        n70 = Initialize Array(0.0 ("element"), w677, 13 ("dimension size")) -> (w676:dbl[][])
        n71 = property class="Globals"(reference=w678, error in=w679, "Properties:C1"=w676, "Properties:C2"=w676, "Properties:C3"=w676, "Properties:C4"=w676, "Properties:C5"=w676, "Properties:C6"=w676, "Properties:C7"=w676, "Properties:C9"=w676) -> (error out=w681:errorcluster)  [unwired: 1 out]
      }
      frame Default {
        # "NO TEST CODE\nAlways dedicate the \"Default\" case to EXIT the Sequencer Loop."
        # "Exit Loop"
      }
    }
    n72 = Or(x=w16, y=w20) -> (x .or. y?=w17:bool)
  }
  "error out" <- w10
  n73 = Unbundle By Name(w2) -> ("Initial Configurations"=→"Initial Configurations":T1)
